vi "home page.vi"() -> ()   [LabVIEW 2019]
uses:
  <vilib>/vision/Image Controls.llb/IMAQ Image.ctl
  <vilib>/Utility/NIReport.llb/Report Type.ctl
  <vilib>/addons/database/Connection.llb/DB Tools Open Connec (String).vi
  <vilib>/addons/_office/excel.llb/Excel Easy Table (str).vi
  <vilib>/measure/mamon.llb/Trigger Detection for 1 Channel.vi
  <vilib>/Utility/NIReport.llb/NI_report.lvclass
  defectsWrapper/defectsWrapper.lvlib
  <vilib>/vision/NI_Vision_Development_Module.lvlib
  <vilib>/vision/driver/NI_Vision_Acquisition_Software.lvlib
  <vilib>/userDefined/High Color/IMAQdx.ctl
  <vilib>/Utility/error.llb/DialogType.ctl
  <vilib>/addons/_office/NI_ReportGenerationToolkit.lvlib
  <vilib>/Utility/NIReport.llb/NI_ReportGenerationCore.lvlib
  <vilib>/measure/NI_MAPro.lvlib
  <vilib>/addons/database/NI_Database_API.lvlib
panel:
  out "sensor thr array":dbl[](array[numeric])
  out "info array":dbl[][](array[numeric])
  out "process error out  2":errorcluster
  out "nan error num":i32
  out "alarm error":errorcluster
  out "sensor error out":errorcluster
  out "img show error":errorcluster
  out "query error in":errorcluster
  out "camera error out":errorcluster
  out "sensor error in":errorcluster
  out "rotate array":errorcluster[](array[cluster])
  out "camera error in":errorcluster
  out "calibration error":errorcluster
  out "rotate error":errorcluster
  out "all errors":errorcluster
  out "DB days to save":i16
  out "orgin data":dbl[](array[numeric])
  out "last difrence":i16
  out "stop ok 2":bool caption="OK"
  out "Overal CURV avg(mm)":dbl format="%#_2g"
  out "Debounce Time":dbl
  out "Frame False Thr":dbl
  out "Col Curves":dbl[](array[numeric])
  out "bottum loop stop":bool
  out "coloumn count stop":bool
  out "query stop":bool=TRUE
  out "alarm loop stop":bool=TRUE
  out "setting stop":bool
  out "rotate stop":bool=TRUE
  out "selected pallet stop":bool
  out "database name":string
  out "denois level array":dbl[](array[numeric])
  out "falling level thr":dbl=59000.0 format="%#_13g"
  out "rotate":bool=TRUE
  out "sen plt indx":i32
  out "snap img":T1
  out "Proc":bool
  out "Frm False":bool
  out "Run/Stop":bool
  out "Sync":bool
  out "Speed (m/min)":string="0"
  out "PLT NUM :":string="1"
  out "avg data array":dbl[](array[numeric])
  out "curv sw info":dbl[](array[numeric])
  out "stop ok":bool caption="OK"
  out "stop live view":bool
  out "stop tab control":bool
  out "dis plt number":i32=45
  out "Tabe name":string="pallet"
  out "PLT NUM":i16
  out "time&date 2":string="08:00:00"
  out "time&date":string="2020/11/22"
  in  "Home":bool
  out "Plt Count":bool
  out "Col. Count":bool
  in  "Sequence Button":bool
  in  "setting":bool
  in  "Graph Button":bool
  in  "report":bool
  in  "stop 3":bool
  out "DPIS":string="DPIS"
  out "capture or not?":bool=TRUE
  out "ready":bool
  out "capture triger":bool
  out "sensor counter":bool
  out "alarm edge":bool
  out "alarm":bool
  out "BoolText.Text":string
  out "counting role":T2(ring)
  out "ch sw sensor2":dbl
  out "ch sw sensor1":dbl
  out "ch sensor3":dbl
  out "ch sensor2":dbl
  out "ch sensor1":dbl
  out "timout":u32=50
  out "Remote Port":u16=502
  out "IP #":string="192.168.88.7"
  out "threshoulds":dbl[](array[numeric])=[900.0, 1000.0, 1600.0, 2400.0, 3000.0, 3000.0]
  out "1st thr":dbl=25.0
  out "2nd thr":dbl=50.0
  out "1st sensor thr":u32=26500
  out "2nd sensor thr":u16=30000
  out "3rd sensor thr":u16=30000
  out "size":dbl=5.0
  out "path image":path
  in  "Button":bool
  out "initilized array":i16[](array[numeric])
  out "Tab Control":enum32{"Page 1", "Page 2", "Page 3"}(tab)
  in  "capture":bool
  out "speed 2":dbl
  out "DEF Type":dbl format="%#.1g"
  out "Sen Plt\nNUM":i16
  out "CURV (mm)":dbl format="%#_3g"
  out "GB defects%":dbl format="%#.1g"
  out "Alarm":bool
  in  "OFF":bool
  out "Pallet Defects View":T1(plugin-control)
  out "GB sit":u32(colorbox)=16448250
  out "curv sit":bool
  out "SWR 2":bool
  out "SWL 2":bool
  in  "Refresh Button":bool
  in  "PLT NUM SYNC":i16
  out "Col\n NUM":dbl format="%#.1g"
  out "Live View":T1(plugin-control)
  out "Col5 CURV(mm)":dbl format="%#_2g"
  out "Sensor Pallet NUM":i16
  out "SideWall Sensors Graph":dynamicdata(graph)=[{"t0"=timestamp(3688782360.9322495 s since 1904-01-01), "dt"=1.0, "Y"=[6594.0]}, {"t0"=timestamp(3688782360.9322495 s since 1904-01-01), "dt"=1.0, "Y"=[65535.0]}]
  out "Col1 CURV(mm)":dbl format="%#_2g"
  out "Col2 CURV(mm)":dbl format="%#_2g"
  out "Col3 CURV(mm)":dbl format="%#_2g"
  out "Col4 CURV(mm)":dbl format="%#_2g"
  out "Overal CURV(mm)":dbl format="%#_2g"
  out "Curvness Sensors Graph":dynamicdata(graph)
  in  "Search Button 2":bool
  in  "Save As Button 2":bool
  in  "pallet sit sel":bool
  in  "swl sel":bool
  in  "swr sel":bool
  in  "PALLET SITUATION":u16(ring) items=["Normal", "Warning", "Error"]
  in  "SWL":u16(ring) items=["Normal", "Error"]
  in  "SWR":u16(ring) items=["Normal", "Error"]
  in  "curv sit sel":bool
  in  "CURV SITUATION":u16(ring) items=["Normal", "Error"]
  in  "def type sel":bool
  in  "DEFECTS TYPE":u16(ring) items=["1", "2"]
  in  "GB_sit sel":bool
  in  "GB SITUATION":u16(ring) items=["Normal", "Warning", "Error"]
  in  "UNTIL":timestamp format="%<%X\n%x>T"
  in  "FROM":timestamp format="%<%X\n%x>T"
  in  "plt num sel":bool
  in  "PALLET NUMBER":dbl
  in  "time sel":bool=TRUE
  in  "TIME":u16(ring)=4 items=["Selected Period", "Last Day", "Last Week", "Last Mounth", "Last Turn"]
  out "Table":string[][](table)
  in  "Base Path":path=path "C:/excel files"
  out "bottum array":bool[](array[boolean])
  out "bottum refrence":refnum<vi>[](array[refnum])
  out "bt ref array":refnum<vi>[](array[refnum])
  in  "117":bool
  in  "118":bool
  in  "119":bool
  in  "120":bool
  in  "121":bool
  in  "122":bool
  in  "123":bool
  in  "124":bool
  in  "125":bool
  in  "126":bool
  in  "127":bool
  in  "128":bool
  in  "129":bool
  in  "130":bool
  in  "131":bool
  in  "132":bool
  in  "133":bool
  in  "134":bool
  in  "135":bool
  in  "136":bool
  in  "137":bool
  in  "138":bool
  in  "139":bool
  in  "140":bool
  in  "141":bool
  in  "142":bool
  in  "143":bool
  in  "144":bool
  in  "145":bool
  in  "146":bool
  in  "147":bool
  in  "148":bool
  in  "149":bool
  in  "150":bool
  in  "151":bool
  in  "152":bool
  in  "153":bool
  in  "154":bool
  in  "155":bool
  in  "156":bool
  in  "157":bool
  in  "158":bool
  in  "159":bool
  in  "160":bool
  in  "161":bool
  in  "162":bool
  in  "163":bool
  in  "164":bool
  in  "165":bool
  in  "166":bool
  in  "167":bool
  in  "168":bool
  in  "169":bool
  in  "170":bool
  in  "171":bool
  in  "172":bool
  in  "173":bool
  in  "174":bool
  in  "175":bool
  in  "176":bool
  in  "177":bool
  in  "178":bool
  in  "179":bool
  in  "180":bool
  in  "181":bool
  in  "182":bool
  in  "183":bool
  in  "184":bool
  in  "185":bool
  in  "186":bool
  in  "187":bool
  in  "188":bool
  in  "189":bool
  in  "190":bool
  in  "191":bool
  in  "192":bool
  in  "193":bool
  in  "194":bool
  in  "195":bool
  in  "196":bool
  in  "197":bool
  in  "198":bool
  in  "199":bool
  in  "200":bool
  in  "201":bool
  in  "202":bool
  in  "203":bool
  in  "204":bool
  in  "205":bool
  in  "206":bool
  in  "207":bool
  in  "208":bool
  in  "209":bool
  in  "210":bool
  in  "211":bool
  in  "212":bool
  in  "213":bool
  in  "214":bool
  in  "215":bool
  in  "216":bool
  in  "217":bool
  in  "218":bool
  in  "219":bool
  in  "220":bool
  in  "221":bool
  in  "222":bool
  in  "223":bool
  in  "224":bool
  in  "225":bool
  in  "226":bool
  in  "227":bool
  in  "228":bool
  in  "229":bool
  in  "230":bool
  in  "231":bool
  in  "232":bool
  in  "116":bool
  in  "115":bool
  in  "114":bool
  in  "113":bool
  in  "112":bool
  in  "111":bool
  in  "110":bool
  in  "109":bool
  in  "108":bool
  in  "107":bool
  in  "106":bool
  in  "105":bool
  in  "104":bool
  in  "103":bool
  in  "102":bool
  in  "101":bool
  in  "100":bool
  in  "99":bool
  in  "98":bool
  in  "97":bool
  in  "96":bool
  in  "95":bool
  in  "94":bool
  in  "93":bool
  in  "92":bool
  in  "91":bool
  in  "90":bool
  in  "89":bool
  in  "88":bool
  in  "87":bool
  in  "86":bool
  in  "85":bool
  in  "84":bool
  in  "83":bool
  in  "82":bool
  in  "81":bool
  in  "80":bool
  in  "79":bool
  in  "78":bool
  in  "77":bool
  in  "76":bool
  in  "75":bool
  in  "74":bool
  in  "73":bool
  in  "72":bool
  in  "71":bool
  in  "70":bool
  in  "69":bool
  in  "68":bool
  in  "67":bool
  in  "66":bool
  in  "65":bool
  in  "64":bool
  in  "63":bool
  in  "62":bool
  in  "61":bool
  in  "60":bool
  in  "59":bool
  in  "58":bool
  in  "57":bool
  in  "56":bool
  in  "55":bool
  in  "54":bool
  in  "53":bool
  in  "52":bool
  in  "51":bool
  in  "50":bool
  in  "49":bool
  in  "48":bool
  in  "47":bool
  in  "46":bool
  in  "45":bool
  in  "44":bool
  in  "43":bool
  in  "42":bool
  in  "41":bool
  in  "40":bool
  in  "39":bool
  in  "38":bool
  in  "37":bool
  in  "36":bool
  in  "35":bool
  in  "34":bool
  in  "33":bool
  in  "32":bool
  in  "31":bool
  in  "30":bool
  in  "29":bool
  in  "28":bool
  in  "27":bool
  in  "26":bool
  in  "25":bool
  in  "24":bool
  in  "23":bool
  in  "22":bool
  in  "21":bool
  in  "20":bool
  in  "19":bool
  in  "18":bool
  in  "17":bool
  in  "16":bool
  in  "15":bool
  in  "14":bool
  in  "13":bool
  in  "12":bool
  in  "11":bool
  in  "10":bool
  in  "9":bool
  in  "8":bool
  in  "7":bool
  in  "6":bool
  in  "5":bool
  in  "4":bool
  in  "3":bool
  in  "2":bool
  in  "1":bool
types:
  T1 = typedef "IMAQ Image.ctl" = refnum<image>
  T2 = enum16{"1st sensor", "2nd sensor", "3rd sensor", "1st+2nd", "1st+3rd", "2nd+3rd", "1st+2nd+3rd"}
  T3 = typedef "Image Type" = u32
  T4 = typedef "IMAQdx.ctl" = refnum<k21>
  T5 = typedef "DialogType.ctl" = u16
  T6 = enum8{"Enabled", "Disabled", "Disabled and Grayed Out"}
  T7 = typedef "NI_Database_API.lvlib/Conn ObjectReference.ctl" = refnum<k1>
  T8 = cluster{"ch sensor1":dbl, "ch sensor2":dbl, "ch sensor3":dbl, "ch sw sensor1":dbl, "ch sw sensor2":dbl}
  T9 = enum32{"Invalid", "Standard", "Closed", "Hidden", "Minimized", "Maximized"}
  T10 = cluster{"ch sensor1":dbl, "ch sensor2":dbl, "chs ensor3":dbl, "ch sw sensor1":dbl, "ch sw sensor2":dbl}
  T11 = cluster{"level1 thr":dbl, "level2 thr":dbl, "gr.th1":dbl, "gr.th2":dbl, "gr.th3":dbl, "gr.th4":dbl, "gr.th5":dbl, "gr.th6":dbl, "gr.th7":dbl, "gr.th8":dbl, "gr.th9":dbl, "def size":dbl, "Frame False Thr":dbl}
  T12 = cluster{"Thr1":dbl, "Thr2":dbl, "Thr3":dbl, "Port":dbl, "time out":dbl, "SWR thr":dbl, "SWL thr ":dbl, "Curv thr (mm)":dbl, "SW timout(s)":dbl, "falling level thr":dbl, "denoise thr1":dbl, "denoise thr2":dbl, "denoise thr3":dbl, "low level read thr":dbl, "Debounce Time":dbl}
  T13 = cluster{"plt number dis":i16, "Table Name":string, "Database Name":string, "DB days to save":i16}
  T14 = enum16{"maximized", "minimized", "normal", "no change"}
  T15 = typedef "NI_ReportGenerationCore.lvlib/Report Type.ctl" = enum16{"HTML", "Word", "Excel"}
  T16 = typedef "LVDateTimeRec.ctl" = cluster{"fractional second":dbl, "second":i32, "minute":i32, "hour":i32, "day of month":i32, "month":i32, "year":i32, "day of week":i32, "day of year":i32, "DST":i32}
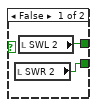
[diagram p6: hidden frame]
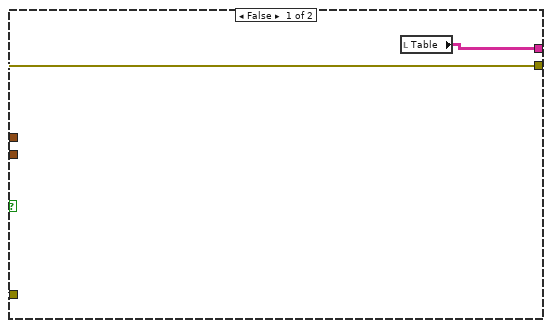
[diagram p8: hidden frame]
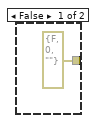
[diagram p10: hidden frame]
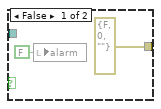
[diagram p11: hidden frame]
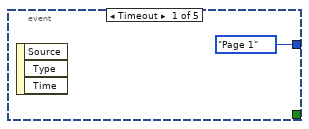
[diagram p14: hidden frame]
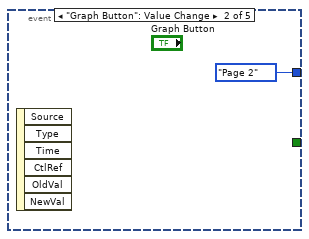
[diagram p15: hidden frame]
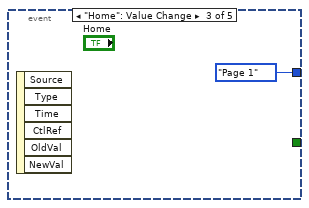
[diagram p16: hidden frame]
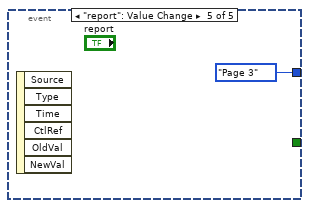
[diagram p17: hidden frame]
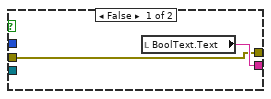
[diagram p19: hidden frame]
diagram:
  w26 = 2 ("dimension size")
  w21 = 100 ("dimension size")
  (unwired) FALSE ("process")
  w67 = FALSE ("nan error")
  w68 = 0.0
  w75 = FALSE
  w100 = T3 4 items=["Grayscale (U8)", "Grayscale (I16)", "Grayscale (SGL)", "Complex (CSG)", "RGB (U32)", "HSL (U32)", "RGB (U64)", "Grayscale (U16)"] ("Image Type")
  n1 = call "load Defects Script.vi"() -> ()  [unwired: 11 in, 1 out]
  n2 = while {
    tunnel: [w345] -> w62
    stop <- w345 stop-if-true
    n3 = Wait (ms)(milliseconds to wait=u32 5) -> ()  [unwired: 1 out]
    n4 = local read "stop ok"() -> (w345:bool)
    n5 = Build Array("232", "231", "230", "229", "228", "227", "226", "225", "224", "223", "222", "221", "220", "219", "218", "217", "216", "215", "214", "213", "212", "211", "210", "209", "208", "207", "206", "205", "204", "203", "202", "201", "200", "199", "198", "197", "196", "195", "194", "193", "192", "191", "190", "189", "188", "187", "186", "185", "184", "183", "182", "181", "180", "179", "178", "177", "176", "175", "174", "173", "172", "171", "170", "169", "168", "167", "166", "165", "164", "163", "162", "161", "160", "159", "158", "157", "156", "155", "154", "153", "152", "151", "150", "149", "148", "147", "146", "145", "144", "143", "142", "141", "140", "139", "138", "137", "136", "135", "134", "133", "132", "131", "130", "129", "128", "127", "126", "125", "124", "123", "122", "121", "120", "119", "118", "117", "116", "115", "114", "113", "112", "111", "110", "109", "108", "107", "106", "105", "104", "103", "102", "101", "100", "99", "98", "97", "96", "95", "94", "93", "92", "91", "90", "89", "88", "87", "86", "85", "84", "83", "82", "81", "80", "79", "78", "77", "76", "75", "74", "73", "72", "71", "70", "69", "68", "67", "66", "65", "64", "63", "62", "61", "60", "59", "58", "57", "56", "55", "54", "53", "52", "51", "50", "49", "48", "47", "46", "45", "44", "43", "42", "41", "40", "39", "38", "37", "36", "35", "34", "33", "32", "31", "30", "29", "28", "27", "26", "25", "24", "23", "22", "21", "20", "19", "18", "17", "16", "15", "14", "13", "12", "11", "10", "9", "8", "7", "6", "5", "4", "3", "2", "1") -> (→"bottum array":bool[])
  }
  "bottum loop stop" <- w62
  n6 = control-ref of="232"() -> (w344:refnum<vi>)
  n7 = control-ref of="231"() -> (w343:refnum<vi>)
  n8 = control-ref of="230"() -> (w342:refnum<vi>)
  n9 = control-ref of="229"() -> (w341:refnum<vi>)
  n10 = control-ref of="228"() -> (w340:refnum<vi>)
  n11 = control-ref of="227"() -> (w339:refnum<vi>)
  n12 = control-ref of="226"() -> (w338:refnum<vi>)
  n13 = control-ref of="225"() -> (w337:refnum<vi>)
  n14 = control-ref of="224"() -> (w336:refnum<vi>)
  n15 = control-ref of="223"() -> (w335:refnum<vi>)
  n16 = control-ref of="222"() -> (w334:refnum<vi>)
  n17 = control-ref of="221"() -> (w333:refnum<vi>)
  n18 = control-ref of="220"() -> (w332:refnum<vi>)
  n19 = control-ref of="219"() -> (w331:refnum<vi>)
  n20 = control-ref of="218"() -> (w330:refnum<vi>)
  n21 = control-ref of="217"() -> (w329:refnum<vi>)
  n22 = control-ref of="216"() -> (w328:refnum<vi>)
  n23 = control-ref of="215"() -> (w327:refnum<vi>)
  n24 = control-ref of="214"() -> (w326:refnum<vi>)
  n25 = control-ref of="213"() -> (w325:refnum<vi>)
  n26 = control-ref of="212"() -> (w324:refnum<vi>)
  n27 = control-ref of="211"() -> (w323:refnum<vi>)
  n28 = control-ref of="210"() -> (w322:refnum<vi>)
  n29 = control-ref of="209"() -> (w321:refnum<vi>)
  n30 = control-ref of="208"() -> (w320:refnum<vi>)
  n31 = control-ref of="207"() -> (w319:refnum<vi>)
  n32 = control-ref of="206"() -> (w318:refnum<vi>)
  n33 = control-ref of="205"() -> (w317:refnum<vi>)
  n34 = control-ref of="204"() -> (w316:refnum<vi>)
  n35 = control-ref of="203"() -> (w315:refnum<vi>)
  n36 = control-ref of="202"() -> (w314:refnum<vi>)
  n37 = control-ref of="201"() -> (w313:refnum<vi>)
  n38 = control-ref of="200"() -> (w312:refnum<vi>)
  n39 = control-ref of="199"() -> (w311:refnum<vi>)
  n40 = control-ref of="198"() -> (w310:refnum<vi>)
  n41 = control-ref of="197"() -> (w309:refnum<vi>)
  n42 = control-ref of="196"() -> (w308:refnum<vi>)
  n43 = control-ref of="195"() -> (w307:refnum<vi>)
  n44 = control-ref of="194"() -> (w306:refnum<vi>)
  n45 = control-ref of="193"() -> (w305:refnum<vi>)
  n46 = control-ref of="192"() -> (w304:refnum<vi>)
  n47 = control-ref of="191"() -> (w303:refnum<vi>)
  n48 = control-ref of="190"() -> (w302:refnum<vi>)
  n49 = control-ref of="189"() -> (w301:refnum<vi>)
  n50 = control-ref of="188"() -> (w300:refnum<vi>)
  n51 = control-ref of="187"() -> (w299:refnum<vi>)
  n52 = control-ref of="186"() -> (w298:refnum<vi>)
  n53 = control-ref of="185"() -> (w297:refnum<vi>)
  n54 = control-ref of="184"() -> (w296:refnum<vi>)
  n55 = control-ref of="183"() -> (w295:refnum<vi>)
  n56 = control-ref of="182"() -> (w294:refnum<vi>)
  n57 = control-ref of="181"() -> (w293:refnum<vi>)
  n58 = control-ref of="180"() -> (w292:refnum<vi>)
  n59 = control-ref of="179"() -> (w291:refnum<vi>)
  n60 = control-ref of="178"() -> (w290:refnum<vi>)
  n61 = control-ref of="177"() -> (w289:refnum<vi>)
  n62 = control-ref of="176"() -> (w288:refnum<vi>)
  n63 = control-ref of="175"() -> (w287:refnum<vi>)
  n64 = control-ref of="174"() -> (w286:refnum<vi>)
  n65 = control-ref of="173"() -> (w285:refnum<vi>)
  n66 = control-ref of="172"() -> (w284:refnum<vi>)
  n67 = control-ref of="171"() -> (w283:refnum<vi>)
  n68 = control-ref of="170"() -> (w282:refnum<vi>)
  n69 = control-ref of="169"() -> (w281:refnum<vi>)
  n70 = control-ref of="168"() -> (w280:refnum<vi>)
  n71 = control-ref of="167"() -> (w279:refnum<vi>)
  n72 = control-ref of="166"() -> (w278:refnum<vi>)
  n73 = control-ref of="165"() -> (w277:refnum<vi>)
  n74 = control-ref of="164"() -> (w276:refnum<vi>)
  n75 = control-ref of="163"() -> (w275:refnum<vi>)
  n76 = control-ref of="162"() -> (w274:refnum<vi>)
  n77 = control-ref of="161"() -> (w273:refnum<vi>)
  n78 = control-ref of="160"() -> (w272:refnum<vi>)
  n79 = control-ref of="159"() -> (w271:refnum<vi>)
  n80 = control-ref of="158"() -> (w270:refnum<vi>)
  n81 = control-ref of="157"() -> (w269:refnum<vi>)
  n82 = control-ref of="156"() -> (w268:refnum<vi>)
  n83 = control-ref of="155"() -> (w267:refnum<vi>)
  n84 = control-ref of="154"() -> (w266:refnum<vi>)
  n85 = control-ref of="153"() -> (w265:refnum<vi>)
  n86 = control-ref of="152"() -> (w264:refnum<vi>)
  n87 = control-ref of="151"() -> (w263:refnum<vi>)
  n88 = control-ref of="150"() -> (w262:refnum<vi>)
  n89 = control-ref of="149"() -> (w261:refnum<vi>)
  n90 = control-ref of="148"() -> (w260:refnum<vi>)
  n91 = control-ref of="147"() -> (w259:refnum<vi>)
  n92 = control-ref of="146"() -> (w258:refnum<vi>)
  n93 = control-ref of="145"() -> (w257:refnum<vi>)
  n94 = control-ref of="144"() -> (w256:refnum<vi>)
  n95 = control-ref of="143"() -> (w255:refnum<vi>)
  n96 = control-ref of="142"() -> (w254:refnum<vi>)
  n97 = control-ref of="141"() -> (w253:refnum<vi>)
  n98 = control-ref of="140"() -> (w252:refnum<vi>)
  n99 = control-ref of="139"() -> (w251:refnum<vi>)
  n100 = control-ref of="138"() -> (w250:refnum<vi>)
  n101 = control-ref of="137"() -> (w249:refnum<vi>)
  n102 = control-ref of="136"() -> (w248:refnum<vi>)
  n103 = control-ref of="135"() -> (w247:refnum<vi>)
  n104 = control-ref of="134"() -> (w246:refnum<vi>)
  n105 = control-ref of="133"() -> (w245:refnum<vi>)
  n106 = control-ref of="132"() -> (w244:refnum<vi>)
  n107 = control-ref of="131"() -> (w243:refnum<vi>)
  n108 = control-ref of="130"() -> (w242:refnum<vi>)
  n109 = control-ref of="129"() -> (w241:refnum<vi>)
  n110 = control-ref of="128"() -> (w240:refnum<vi>)
  n111 = control-ref of="127"() -> (w239:refnum<vi>)
  n112 = control-ref of="126"() -> (w238:refnum<vi>)
  n113 = control-ref of="125"() -> (w237:refnum<vi>)
  n114 = control-ref of="124"() -> (w236:refnum<vi>)
  n115 = control-ref of="123"() -> (w235:refnum<vi>)
  n116 = control-ref of="122"() -> (w234:refnum<vi>)
  n117 = control-ref of="121"() -> (w233:refnum<vi>)
  n118 = control-ref of="120"() -> (w232:refnum<vi>)
  n119 = control-ref of="119"() -> (w231:refnum<vi>)
  n120 = control-ref of="118"() -> (w230:refnum<vi>)
  n121 = control-ref of="117"() -> (w229:refnum<vi>)
  n122 = control-ref of="116"() -> (w228:refnum<vi>)
  n123 = control-ref of="115"() -> (w227:refnum<vi>)
  n124 = control-ref of="114"() -> (w226:refnum<vi>)
  n125 = control-ref of="113"() -> (w225:refnum<vi>)
  n126 = control-ref of="112"() -> (w224:refnum<vi>)
  n127 = control-ref of="111"() -> (w223:refnum<vi>)
  n128 = control-ref of="110"() -> (w222:refnum<vi>)
  n129 = control-ref of="109"() -> (w221:refnum<vi>)
  n130 = control-ref of="108"() -> (w220:refnum<vi>)
  n131 = control-ref of="107"() -> (w219:refnum<vi>)
  n132 = control-ref of="106"() -> (w218:refnum<vi>)
  n133 = control-ref of="105"() -> (w217:refnum<vi>)
  n134 = control-ref of="104"() -> (w216:refnum<vi>)
  n135 = control-ref of="103"() -> (w215:refnum<vi>)
  n136 = control-ref of="102"() -> (w214:refnum<vi>)
  n137 = control-ref of="101"() -> (w213:refnum<vi>)
  n138 = control-ref of="100"() -> (w212:refnum<vi>)
  n139 = control-ref of="99"() -> (w211:refnum<vi>)
  n140 = control-ref of="98"() -> (w210:refnum<vi>)
  n141 = control-ref of="97"() -> (w209:refnum<vi>)
  n142 = control-ref of="96"() -> (w208:refnum<vi>)
  n143 = control-ref of="95"() -> (w207:refnum<vi>)
  n144 = control-ref of="94"() -> (w206:refnum<vi>)
  n145 = control-ref of="93"() -> (w205:refnum<vi>)
  n146 = control-ref of="92"() -> (w204:refnum<vi>)
  n147 = control-ref of="91"() -> (w203:refnum<vi>)
  n148 = control-ref of="90"() -> (w202:refnum<vi>)
  n149 = control-ref of="89"() -> (w201:refnum<vi>)
  n150 = control-ref of="88"() -> (w200:refnum<vi>)
  n151 = control-ref of="87"() -> (w199:refnum<vi>)
  n152 = control-ref of="86"() -> (w198:refnum<vi>)
  n153 = control-ref of="85"() -> (w197:refnum<vi>)
  n154 = control-ref of="84"() -> (w196:refnum<vi>)
  n155 = control-ref of="83"() -> (w195:refnum<vi>)
  n156 = control-ref of="82"() -> (w194:refnum<vi>)
  n157 = control-ref of="81"() -> (w193:refnum<vi>)
  n158 = control-ref of="80"() -> (w192:refnum<vi>)
  n159 = control-ref of="79"() -> (w191:refnum<vi>)
  n160 = control-ref of="78"() -> (w190:refnum<vi>)
  n161 = control-ref of="77"() -> (w189:refnum<vi>)
  n162 = control-ref of="76"() -> (w188:refnum<vi>)
  n163 = control-ref of="75"() -> (w187:refnum<vi>)
  n164 = control-ref of="74"() -> (w186:refnum<vi>)
  n165 = control-ref of="73"() -> (w185:refnum<vi>)
  n166 = control-ref of="72"() -> (w184:refnum<vi>)
  n167 = control-ref of="71"() -> (w183:refnum<vi>)
  n168 = control-ref of="70"() -> (w182:refnum<vi>)
  n169 = control-ref of="69"() -> (w181:refnum<vi>)
  n170 = control-ref of="68"() -> (w180:refnum<vi>)
  n171 = control-ref of="67"() -> (w179:refnum<vi>)
  n172 = control-ref of="66"() -> (w178:refnum<vi>)
  n173 = control-ref of="65"() -> (w177:refnum<vi>)
  n174 = control-ref of="64"() -> (w176:refnum<vi>)
  n175 = control-ref of="63"() -> (w175:refnum<vi>)
  n176 = control-ref of="62"() -> (w174:refnum<vi>)
  n177 = control-ref of="61"() -> (w173:refnum<vi>)
  n178 = control-ref of="60"() -> (w172:refnum<vi>)
  n179 = control-ref of="59"() -> (w171:refnum<vi>)
  n180 = local write "capture or not?"(w67) -> ()
  n181 = local write "stop ok"(w67) -> ()
  n182 = local write "alarm"(w67) -> ()
  n183 = property on="Alarm" class="Bool (strict)"() -> ("Colors [4]"=w98:cluster{u32, u32}[])  [unwired: 2 in, 2 out]
  n184 = control-ref of="58"() -> (w170:refnum<vi>)
  n185 = control-ref of="57"() -> (w169:refnum<vi>)
  n186 = control-ref of="56"() -> (w168:refnum<vi>)
  n187 = control-ref of="55"() -> (w167:refnum<vi>)
  n188 = control-ref of="54"() -> (w166:refnum<vi>)
  n189 = control-ref of="53"() -> (w165:refnum<vi>)
  n190 = control-ref of="52"() -> (w164:refnum<vi>)
  n191 = control-ref of="51"() -> (w163:refnum<vi>)
  n192 = control-ref of="50"() -> (w162:refnum<vi>)
  n193 = control-ref of="49"() -> (w161:refnum<vi>)
  n194 = control-ref of="48"() -> (w160:refnum<vi>)
  n195 = control-ref of="47"() -> (w159:refnum<vi>)
  n196 = control-ref of="46"() -> (w158:refnum<vi>)
  n197 = control-ref of="45"() -> (w157:refnum<vi>)
  n198 = control-ref of="44"() -> (w156:refnum<vi>)
  n199 = control-ref of="43"() -> (w155:refnum<vi>)
  n200 = control-ref of="42"() -> (w154:refnum<vi>)
  n201 = control-ref of="41"() -> (w153:refnum<vi>)
  n202 = control-ref of="40"() -> (w152:refnum<vi>)
  n203 = control-ref of="39"() -> (w151:refnum<vi>)
  n204 = control-ref of="38"() -> (w150:refnum<vi>)
  n205 = control-ref of="37"() -> (w149:refnum<vi>)
  n206 = control-ref of="36"() -> (w148:refnum<vi>)
  n207 = control-ref of="35"() -> (w147:refnum<vi>)
  n208 = control-ref of="34"() -> (w146:refnum<vi>)
  n209 = control-ref of="33"() -> (w145:refnum<vi>)
  n210 = control-ref of="32"() -> (w144:refnum<vi>)
  n211 = control-ref of="31"() -> (w143:refnum<vi>)
  n212 = control-ref of="30"() -> (w142:refnum<vi>)
  n213 = control-ref of="29"() -> (w141:refnum<vi>)
  n214 = control-ref of="28"() -> (w140:refnum<vi>)
  n215 = control-ref of="27"() -> (w139:refnum<vi>)
  n216 = control-ref of="26"() -> (w138:refnum<vi>)
  n217 = control-ref of="25"() -> (w137:refnum<vi>)
  n218 = control-ref of="24"() -> (w136:refnum<vi>)
  n219 = control-ref of="23"() -> (w135:refnum<vi>)
  n220 = control-ref of="22"() -> (w134:refnum<vi>)
  n221 = control-ref of="21"() -> (w133:refnum<vi>)
  n222 = control-ref of="20"() -> (w132:refnum<vi>)
  n223 = control-ref of="19"() -> (w131:refnum<vi>)
  n224 = control-ref of="18"() -> (w130:refnum<vi>)
  n225 = control-ref of="17"() -> (w129:refnum<vi>)
  n226 = control-ref of="16"() -> (w128:refnum<vi>)
  n227 = control-ref of="15"() -> (w127:refnum<vi>)
  n228 = control-ref of="14"() -> (w126:refnum<vi>)
  n229 = control-ref of="13"() -> (w125:refnum<vi>)
  n230 = control-ref of="12"() -> (w124:refnum<vi>)
  n231 = control-ref of="11"() -> (w123:refnum<vi>)
  n232 = control-ref of="10"() -> (w122:refnum<vi>)
  n233 = control-ref of="9"() -> (w121:refnum<vi>)
  n234 = control-ref of="8"() -> (w120:refnum<vi>)
  n235 = control-ref of="7"() -> (w119:refnum<vi>)
  n236 = control-ref of="6"() -> (w118:refnum<vi>)
  n237 = control-ref of="5"() -> (w117:refnum<vi>)
  n238 = control-ref of="4"() -> (w116:refnum<vi>)
  n239 = control-ref of="3"() -> (w115:refnum<vi>)
  n240 = control-ref of="2"() -> (w114:refnum<vi>)
  n241 = control-ref of="1"() -> (w113:refnum<vi>)
  n242 = Replace Array Subset(array=w98, new element=cluster{u32, u32} {16448250, 16448250} ("new element/subarray"), index=0) -> (w96:cluster{u32, u32}[])
  n243 = property on="PLT NUM SYNC" class="DigNum (strict)"("Value"=i16 1 ("PLT NUM SYNC")) -> ()  [unwired: 2 in, 2 out]
  n244 = property on="Sen Plt\nNUM" class="DigNum (strict)"("Value"=i16 0 ("Sen Plt\nNUM")) -> ()  [unwired: 2 in, 2 out]
  n245 = property on="GB sit" class="ColBox"("Value"=u32 16448250 ("GB sit")) -> ()  [unwired: 2 in, 2 out]
  n246 = property on="Sensor Pallet NUM" class="DigNum (strict)"("Value"=i16 0 ("Sensor Pallet NUM")) -> ()  [unwired: 2 in, 2 out]
  n247 = property on="Alarm" class="Bool (strict)"("Colors [4]"=w96) -> ()  [unwired: 2 in, 2 out]
  n248 = property on="Col. Count" class="Bool (strict)"("Value"=w75) -> ()  [unwired: 2 in, 2 out]
  n249 = property on="Plt Count" class="Bool (strict)"("Value"=w75) -> ()  [unwired: 2 in, 2 out]
  n250 = property on="Run/Stop" class="Bool (strict)"("Value"=w75) -> ()  [unwired: 2 in, 2 out]
  n251 = property on="curv sit" class="Bool (strict)"("Value"=FALSE ("curv sit")) -> ()  [unwired: 2 in, 2 out]
  n252 = property on="Table" class="Tbl (strict)"("Column Headers[]"=string[] ["PLT_NUM", "DATE_TIME", "GB_DEF", "DEF_TYPE", "GB_SIT", "CURV", "CURV_SIT", "SWR", "SWL", "PLT_SIT", "COL1 CURV", "COL2 CURV", "COL3 CURV", "COL4 CURV", "COL5 CURV"] ("Column Header Strings[]")) -> ()  [unwired: 2 in, 2 out]
  n253 = property on="CURV (mm)" class="DigNum (strict)"("Value"=0.0 ("CURV (mm)")) -> ()  [unwired: 2 in, 2 out]
  n254 = property on="GB defects%" class="DigNum (strict)"("Value"=0.0 ("GB defects%")) -> ()  [unwired: 2 in, 2 out]
  n255 = property on="Speed (m/min)" class="Str"("Value"="0" ("Speed :")) -> ()  [unwired: 2 in, 2 out]
  n256 = property on="time&date 2" class="Str"("Value"="" ("time&date 2")) -> ()  [unwired: 2 in, 2 out]
  n257 = property on="time&date" class="Str"("Value"="" ("time&date")) -> ()  [unwired: 2 in, 2 out]
  n258 = property on="PLT NUM :" class="Str"("Value"="1" ("PLT NUM :")) -> ()  [unwired: 2 in, 2 out]
  n259 = property on="Col\n NUM" class="DigNum (strict)"("Value"=0.0 ("Col\n NUM")) -> ()  [unwired: 2 in, 2 out]
  n260 = property on="DEF Type" class="DigNum (strict)"("Value"=1.0 ("DEF Type")) -> ()  [unwired: 2 in, 2 out]
  n261 = property on="Overal CURV avg(mm)" class="DigNum (strict)"("Value"=0.0 ("Overal CURV(mm)")) -> ()  [unwired: 2 in, 2 out]
  n262 = property on="SWR 2" class="Bool (strict)"("Value"=FALSE ("SWR 2")) -> ()  [unwired: 2 in, 2 out]
  n263 = property on="SWL 2" class="Bool (strict)"("Value"=FALSE ("SWL 2")) -> ()  [unwired: 2 in, 2 out]
  n264 = property on="Proc" class="Bool (strict)"("Value"=FALSE ("Proc")) -> ()  [unwired: 2 in, 2 out]
  n265 = property on="Alarm" class="Bool (strict)"("Blinking"=FALSE ("alarm")) -> ()  [unwired: 2 in, 2 out]
  n266 = property on="Sync" class="Bool (strict)"("Value"=FALSE ("Sync")) -> ()  [unwired: 2 in, 2 out]
  n267 = local write "CURV (mm)"(0.0 ("CURV %")) -> ()
  n268 = property on="Col2 CURV(mm)" class="DigNum (strict)"("Value"=w68) -> ()  [unwired: 2 in, 2 out]
  n269 = property on="Col3 CURV(mm)" class="DigNum (strict)"("Value"=w68) -> ()  [unwired: 2 in, 2 out]
  n270 = property on="Col4 CURV(mm)" class="DigNum (strict)"("Value"=w68) -> ()  [unwired: 2 in, 2 out]
  n271 = property on="Col5 CURV(mm)" class="DigNum (strict)"("Value"=w68) -> ()  [unwired: 2 in, 2 out]
  n272 = property on="Col1 CURV(mm)" class="DigNum (strict)"("Value"=w68) -> ()  [unwired: 2 in, 2 out]
  n273 = Build Array(w344, w343, w342, w341, w340, w339, w338, w337, w336, w335, w334, w333, w332, w331, w330, w329, w328, w327, w326, w325, w324, w323, w322, w321, w320, w319, w318, w317, w316, w315, w314, w313, w312, w311, w310, w309, w308, w307, w306, w305, w304, w303, w302, w301, w300, w299, w298, w297, w296, w295, w294, w293, w292, w291, w290, w289, w288, w287, w286, w285, w284, w283, w282, w281, w280, w279, w278, w277, w276, w275, w274, w273, w272, w271, w270, w269, w268, w267, w266, w265, w264, w263, w262, w261, w260, w259, w258, w257, w256, w255, w254, w253, w252, w251, w250, w249, w248, w247, w246, w245, w244, w243, w242, w241, w240, w239, w238, w237, w236, w235, w234, w233, w232, w231, w230, w229, w228, w227, w226, w225, w224, w223, w222, w221, w220, w219, w218, w217, w216, w215, w214, w213, w212, w211, w210, w209, w208, w207, w206, w205, w204, w203, w202, w201, w200, w199, w198, w197, w196, w195, w194, w193, w192, w191, w190, w189, w188, w187, w186, w185, w184, w183, w182, w181, w180, w179, w178, w177, w176, w175, w174, w173, w172, w171, w170, w169, w168, w167, w166, w165, w164, w163, w162, w161, w160, w159, w158, w157, w156, w155, w154, w153, w152, w151, w150, w149, w148, w147, w146, w145, w144, w143, w142, w141, w140, w139, w138, w137, w136, w135, w134, w133, w132, w131, w130, w129, w128, w127, w126, w125, w124, w123, w122, w121, w120, w119, w118, w117, w116, w115, w114, w113) -> (w109:refnum<vi>[])
  "bottum refrence" <- w109
  n274 = disable-structure shown="Disabled" {
    frame Disabled {
      n275 = call "IMAQ Create"("Image Name"="mainimg", "error in (no error)"=errorcluster {"status"=FALSE, "code"=0, "source"=""}) -> ("New Image"=w593:T1, "error out"=w587:errorcluster)  [unwired: 3 in]
      n276 = call "Vision Acquisition2"("error in"=w587) -> ("Image Out"=w585:T1, "error out"=w582:errorcluster)  [unwired: 24 in, 1 out]
      n277 = call "IMAQ Create"("Image Name"="rotate", "error in (no error)"=w582) -> ("New Image"=w583:T1, "error out"=w581:errorcluster)  [unwired: 3 in]
      n278 = while {
        tunnel: w593 -> [w607]
        tunnel: [w612] -> w590
        tunnel: [w598] -> w588
        tunnel: T4 "cam0" ("Session In") -> [w611]
        tunnel: w585 -> [w610]
        tunnel: w583 -> [w608]
        shift-right: [w599] -> w580
        shift-left: w581 -> [w609]
        stop <- w612 stop-if-true
        # "Live view"
        n279 = flat-sequence {
          tunnel: w611 -> [w620]
          tunnel: w610 -> [w619]
          tunnel: w609 -> [w618]
          tunnel: w608 -> [w615]
          tunnel: w607 -> [w614]
          tunnel: [w617] -> w606
          tunnel: [w616] -> w605
          tunnel: [w615] -> w604
          tunnel: [w614] -> w603
          tunnel: w606 -> [w622]
          tunnel: w605 -> [w623]
          tunnel: w604 -> [w627]
          tunnel: w603 -> [w624]
          tunnel: [w627] -> w602
          tunnel: [w626] -> w601
          tunnel: [w621] -> w600
          tunnel: [w621] -> w595
          tunnel: w602 -> [w630]
          tunnel: w601 -> [w632]
          tunnel: w600 -> [w631]
          tunnel: [w633] -> w597
          tunnel: [w629] -> w596
          tunnel: w595 -> [w628]
          tunnel: [w634] -> w598
          tunnel: [w635] -> w599
          tunnel: w596 -> [w634]
          tunnel: w597 -> [w635]
          frame #0 {
            n280 = call <vilib>:"IMAQdx Grab.vi"("error in"=w618, "Image In"=w619, "Session In"=w620) -> ("error out"=w617:errorcluster, "Image Out"=w616:T1)  [unwired: 1 in, 6 out]
          }
          frame #1 {
            n281 = call "IMAQ Rotate"("error in (no error)"=w622, "Angle (degrees)"=sgl 180.0, "Image Dst"=w624, "Image Src"=w623) -> ("error out"=w626:errorcluster, "Image Dst Out"=w621:T1)  [unwired: 6 in]
          }
          frame #2 {
            n282 = call "IMAQ Copy"("error in (no error)"=w632, "Image Dst"=w630, "Image Src"=w631) -> ("error out"=w633:errorcluster, "Image Dst Out"=w629:T1)  [unwired: 3 in]
            "Live View" <- w628
          }
          frame #3 {
            "snap img" <- w634
          }
        }
        n283 = Wait (ms)(milliseconds to wait=u32 20) -> ()  [unwired: 1 out]
        n284 = local read "stop ok"() -> (w612:bool)
        "camera error in" <- w599
      }
      "stop live view" <- w590
      n285 = call "IMAQ Dispose"("All Images? (No)"=TRUE, "Image"=w588, "error in (no error)"=w580) -> ("error out"=→"camera error out":errorcluster)  [unwired: 3 in]
    }
    frame Enabled {
    }
  }
  n286 = Initialize Array(i16 0 ("element"), 232 ("dimension size")) -> (w110:i16[])
  n287 = property on="Frm False" class="Bool (strict)"("Value"=FALSE ("Frm False")) -> ()  [unwired: 2 in, 2 out]
  n288 = disable-structure shown="Disabled" {
    disable-tunnel: [w638 _] -> w37
    disable-tunnel: [w636 _] -> w18
    frame Disabled {
      n289 = while {
        tunnel: [w652] -> w638
        shift-right: [w639] -> w636
        shift-left: errorcluster {"status"=FALSE, "code"=0, "source"=""} ("error in (no error)") -> [w649]
        stop <- w640 stop-if-true
        w645 = T5 0 items=["no dialog", "OK message", "continue or stop message", "OK message + warnings", "continue/stop + warnings"] ("type of dialog (OK msg:1)")
        n290 = Wait (ms)(milliseconds to wait=u32 5) -> ()  [unwired: 1 out]
        n291 = property on="IP #" class="Str"(error in=w649) -> (error out=w648:errorcluster, "Value"=w651:string)  [unwired: 1 in, 1 out]
        n292 = property on="Remote Port" class="DigNum (strict)"(error in=w648) -> (error out=w647:errorcluster, "Value"=w650:u16)  [unwired: 1 in, 1 out]
        n293 = local read "stop ok"() -> (w641:bool)
        n294 = TCP Open Connection(address=w651, remote port or service name=w650, error in (no error)=w647) -> (connection ID=w652:refnum<k5>, error out=w646:errorcluster)  [unwired: 2 in]
        n295 = call <vilib>:"Simple Error Handler.vi"("type of dialog (OK msg:1)"=w645, "error in (no error)"=w646) -> ("error?"=w644:bool, "error out"=w639:errorcluster)  [unwired: 3 in, 3 out]
        n296 = Not(x=w644) -> (.not. x?=w642:bool)
        n297 = Or(x=w642, y=w641) -> (x .or. y?=w640:bool)
      }
    }
    frame Enabled {
    }
  }
  n298 = for {
    tunnel: [w654] -> w105 mode=indexing
    shift-right: [w664] -> _
    shift-left: w110 -> [w665]
    tunnel: w109 -> [w660] mode=indexing
    tunnel: errorcluster {"status"=FALSE, "code"=0, "source"=""} ("error in (no error)") -> [w659]
    tunnel: [w653] -> w107 mode=indexing
    i -> [w663]
    n299 = Replace Array Subset(array=w665, new element=w663, index=w663) -> (w664:i16[])
    "initilized array" <- w664
    n300 = property class="Bool"(reference=w660, error in=w659) -> (reference out=w669:refnum<vi>, error out=w667:errorcluster, "Label.Text"=w668:string)
    n301 = control-ref of="Button"() -> (w662:refnum<vi>)
    n302 = property class="Bool"(reference=w669, error in=w667, "BoolText.Text"=w668) -> (reference out=w657:refnum<vi>, error out=w658:errorcluster)
    n303 = property class="Bool"(reference=w662) -> ("Colors [4]"=w661:cluster{u32, u32}[])  [unwired: 1 in, 2 out]
    n304 = property class="Bool"(reference=w657, error in=w658, "Colors [4]"=w661) -> (reference out=w656:refnum<vi>, error out=w655:errorcluster)
    n305 = property class="Bool"(reference=w656, error in=w655, "DisabledEnum"=T6."Disabled and Grayed Out" ("Disabled")) -> (reference out=w654:refnum<vi>, error out=w653:errorcluster)
  }
  n306 = Initialize Array(0.0 ("element"), w21) -> (w31:dbl[])
  n307 = Initialize Array(0.0 ("element"), w21) -> (w29:dbl[])
  n308 = Initialize Array(0.0 ("element"), w26) -> (w28:dbl[])
  n309 = Initialize Array(0.0 ("element"), w21) -> (w30:dbl[])
  n310 = Initialize Array(0.0 ("element"), w26) -> (w27:dbl[])
  n311 = call-poly <vilib>:"DB Tools Open Connection.vi"("error in (no error)"=errorcluster {"status"=FALSE, "code"=0, "source"=""}, "connection information"="DSGS" ("database name 2")) -> ("error out"=w48:errorcluster, "connection reference"=w47:T7)  [unwired: 6 in]
  n312 = while {
    tunnel: [w674] -> w92
    tunnel: FALSE ("stop 4") -> [w673]
    tunnel: [FALSE ("Sync")] -> w91
    tunnel: [i16 1 ("PLT NUM SYNC")] -> w90
    stop <- w674 stop-if-true
    # "Tab control"
    n313 = event shown="[3] \"stop 3\": Value Change" {
      selector: _ -> [_ _ _ _ _]
      dyn-events: _ -> [_ _ _ _ _]
      timeout: _ -> [_ _ _ _ _]
      tunnel: [enum32{"Page 1", "Page 2", "Page 3"}."Page 1" ("Tab Control") enum32{"Page 1", "Page 2", "Page 3"}."Page 2" ("Tab Control") enum32{"Page 1", "Page 2", "Page 3"}."Page 1" ("Tab Control") w679 enum32{"Page 1", "Page 2", "Page 3"}."Page 3" ("Tab Control")] -> w670
      tunnel: [_ _ _ w680 _] -> w674
      event Timeout {
        n314 = event-data() -> ()  [unwired: 1 in, 3 out]
      }
      event "Graph Button": Value Change {
        n315 = event-data() -> ()  [unwired: 1 in, 6 out]
      }
      event "Home": Value Change {
        n316 = event-data() -> ()  [unwired: 1 in, 6 out]
      }
      event "stop 3": Value Change {
        n317 = event-data() -> ()  [unwired: 1 in, 6 out]
        n318 = call "close.vi"("Enable"="stop 3") -> ("YES"=w680:bool)  [unwired: 17 in, 1 out]
        "stop ok" <- w680
        n319 = property on="Tab Control" class="TabCtl (strict)"() -> ("Value"=w679:enum32{"Page 1", "Page 2", "Page 3"})  [unwired: 2 in, 2 out]
      }
      event "report": Value Change {
        n320 = event-data() -> ()  [unwired: 1 in, 6 out]
      }
    }
    "Tab Control" <- w670
    n321 = local write "stop tab control"(w673) -> ()
    n322 = Wait (ms)(milliseconds to wait=u32 10) -> ()  [unwired: 1 out]
  }
  "stop tab control" <- w92
  n323 = call "IMAQ Create"("Image Name"="img crop", "error in (no error)"=w48) -> ("New Image"=w55:T1, "error out"=w57:errorcluster)  [unwired: 3 in]
  n324 = local write "PLT NUM SYNC"(w90) -> ()
  n325 = local write "Sync"(w91) -> ()
  n326 = call "IMAQ Create"("Image Name"="pic2", "Image Type"=w100, "error in (no error)"=errorcluster {"status"=FALSE, "code"=0, "source"=""}) -> ("New Image"=w104:T1, "error out"=w103:errorcluster)  [unwired: 2 in]
  n327 = while {
    tunnel: w57 -> [w687]
    tunnel: [w683] -> w54
    stop <- w684 stop-if-true
    n328 = call "load Defects Script.vi"("error in (no error)"=w687) -> ("error out"=w683:errorcluster)  [unwired: 10 in]
    n329 = local read "stop ok"() -> (w685:bool)
    n330 = Not(x=w683) -> (.not. x?=w686:bool)
    n331 = Or(x=w686, y=w685) -> (x .or. y?=w684:bool)
  }
  n332 = while {
    tunnel: w37 -> [w786]
    shift-right: [w767] -> _
    shift-left: w31 -> [w783]
    shift-right: [w762] -> _
    shift-left: w30 -> [w780]
    shift-right: [w761] -> _
    shift-left: w29 -> [w778]
    shift-right: [w760] -> _
    shift-left: w28 -> [w776]
    shift-right: [w759] -> _
    shift-left: w27 -> [w774]
    tunnel: w26 -> [w772]
    shift-right: [w744] -> _
    shift-left: 0.0 ("element") -> [w758]
    tunnel: [w740] -> w24
    tunnel: [FALSE ("Col. Count")] -> w23
    tunnel: [FALSE ("Plt Count")] -> w22
    tunnel: w21 -> [w722]
    tunnel: [w720] -> w20
    shift-right: [w696] -> w19
    shift-left: w18 -> [w785]
    stop <- w720 stop-if-true
    # "coloumn counting"
    n333 = flat-sequence {
      tunnel: w786 -> [w811]
      tunnel: w785 -> [w810]
      tunnel: [w803] -> w784
      tunnel: w783 -> [w802]
      tunnel: [w802] -> w782
      tunnel: [w801] -> w781
      tunnel: w780 -> [w801]
      tunnel: [w800] -> w779
      tunnel: w778 -> [w800]
      tunnel: [w799] -> w777
      tunnel: w776 -> [w799]
      tunnel: [w798] -> w775
      tunnel: w774 -> [w798]
      tunnel: [w797] -> w773
      tunnel: w772 -> [w797]
      tunnel: [w789] -> w771
      tunnel: [w792] -> w770
      tunnel: w758 -> [w796]
      tunnel: [w796] -> w756
      tunnel: [w795] -> w741
      tunnel: [w794] -> w724
      tunnel: [w791] -> w723
      tunnel: w722 -> [w791]
      tunnel: w784 -> [w837]
      tunnel: w782 -> [w836]
      tunnel: w781 -> [w835]
      tunnel: w779 -> [w834]
      tunnel: w777 -> [w833]
      tunnel: w775 -> [w832]
      tunnel: w773 -> [w821]
      tunnel: w771 -> [w831]
      tunnel: w770 -> [w830]
      tunnel: [w817] -> w769
      tunnel: [w818] -> w768
      tunnel: [w829] -> w766
      tunnel: [w828] -> w765
      tunnel: [w827] -> w764
      tunnel: [w826] -> w763
      tunnel: [w825] -> w757
      tunnel: w756 -> [w825]
      tunnel: [w824] -> w755
      tunnel: [w823] -> w742
      tunnel: w741 -> [w823]
      tunnel: w724 -> [w822]
      tunnel: w723 -> [w820]
      tunnel: w769 -> [w857]
      tunnel: w768 -> [w864]
      tunnel: w766 -> [w863]
      tunnel: w765 -> [w862]
      tunnel: w764 -> [w861]
      tunnel: w763 -> [w860]
      tunnel: w757 -> [w858]
      tunnel: w755 -> [w840]
      tunnel: [w864] -> w754
      tunnel: [w863] -> w753
      tunnel: [w862] -> w752
      tunnel: [w861] -> w751
      tunnel: [w860] -> w750
      tunnel: [w857] -> w749
      tunnel: [w856] -> w748
      tunnel: [w846] -> w747
      tunnel: [w855] -> w746
      tunnel: [w854] -> w745
      tunnel: [w853] -> w743
      tunnel: w742 -> [w853]
      tunnel: [w852] -> w738
      tunnel: "capture" -> [w850]
      tunnel: [w843] -> w734
      tunnel: [w842] -> w733
      tunnel: w738 -> [w872]
      tunnel: w743 -> [w876]
      tunnel: "capture" -> [w875]
      tunnel: w745 -> [w873]
      tunnel: w746 -> [w874]
      tunnel: w747 -> [_]
      tunnel: w748 -> [w877]
      tunnel: w749 -> [w870]
      tunnel: w750 -> [w879]
      tunnel: w751 -> [w880]
      tunnel: w752 -> [w881]
      tunnel: w753 -> [w882]
      tunnel: w754 -> [w883]
      tunnel: w734 -> [w869]
      tunnel: w733 -> [w868]
      tunnel: [w883] -> w719
      tunnel: [w882] -> w717
      tunnel: [w881] -> w715
      tunnel: [w880] -> w713
      tunnel: [w879] -> w711
      tunnel: [w871] -> w709
      tunnel: [w873] -> w707
      tunnel: [w876] -> w705
      tunnel: [w868] -> w703
      tunnel: [w868] -> w701
      tunnel: w719 -> [w895]
      tunnel: [w895] -> w718
      tunnel: w717 -> [w894]
      tunnel: [w894] -> w716
      tunnel: w715 -> [w893]
      tunnel: [w893] -> w714
      tunnel: w713 -> [w892]
      tunnel: [w892] -> w712
      tunnel: w711 -> [w891]
      tunnel: [w891] -> w710
      tunnel: w709 -> [w890]
      tunnel: [w890] -> w708
      tunnel: w707 -> [w889]
      tunnel: [w889] -> w706
      tunnel: w705 -> [w888]
      tunnel: [w888] -> w704
      tunnel: w703 -> [w887]
      tunnel: [w887] -> w702
      tunnel: w701 -> [w884]
      tunnel: w718 -> [w908]
      tunnel: w716 -> [w907]
      tunnel: w714 -> [w906]
      tunnel: w712 -> [w905]
      tunnel: w710 -> [w904]
      tunnel: w708 -> [w903]
      tunnel: w706 -> [w902]
      tunnel: w704 -> [w901]
      tunnel: [w908] -> w732
      tunnel: [w907] -> w731
      tunnel: [w906] -> w730
      tunnel: [w905] -> w729
      tunnel: [w904] -> w728
      tunnel: [w903] -> w727
      tunnel: [w902] -> w726
      tunnel: [w901] -> w725
      tunnel: w702 -> [w900]
      tunnel: [w900] -> w721
      tunnel: w721 -> [w912]
      tunnel: w725 -> [w913]
      tunnel: w726 -> [w914]
      tunnel: w727 -> [w915]
      tunnel: w728 -> [w916]
      tunnel: w729 -> [w917]
      tunnel: w730 -> [w918]
      tunnel: w731 -> [w919]
      tunnel: w732 -> [w920]
      tunnel: [w920] -> w695
      tunnel: [w919] -> w694
      tunnel: [w918] -> w693
      tunnel: [w917] -> w692
      tunnel: [w916] -> w691
      tunnel: [w915] -> w690
      tunnel: [w914] -> w689
      tunnel: [w913] -> w688
      tunnel: [w922] -> w740
      tunnel: [w923] -> w696
      tunnel: [w924] -> w744
      tunnel: [w925] -> w759
      tunnel: [w926] -> w760
      tunnel: [w927] -> w761
      tunnel: [w928] -> w762
      tunnel: [w929] -> w767
      tunnel: w695 -> [w929]
      tunnel: w694 -> [w928]
      tunnel: w693 -> [w927]
      tunnel: w692 -> [w926]
      tunnel: w691 -> [w925]
      tunnel: w690 -> [w924]
      tunnel: w689 -> [w923]
      tunnel: w688 -> [w922]
      frame #0 {
        n334 = disable-structure shown="Disabled" {
          disable-tunnel: w811 -> [w816 _]
          disable-tunnel: w810 -> [w815 _]
          disable-tunnel: [w814 _] -> _
          disable-tunnel: [w813 _] -> w795
          disable-tunnel: [w812 _] -> w793
          frame Disabled {
            n335 = call "adamread.vi"("TCP Connection Refnum in"=w816, "error in (no error)"=w815) -> ("TCP Connection Refnum (dup)"=w813:refnum<k5>, "Slave Input Registers 2"=w814:dbl[], "error out 2"=w812:errorcluster)  [unwired: 11 in]
          }
          frame Enabled {
          }
        }
        n336 = local read "ch sensor1"() -> (w804:dbl)
        n337 = local read "ch sensor2"() -> (w805:dbl)
        n338 = local read "ch sensor3"() -> (w806:dbl)
        n339 = local read "ch sw sensor1"() -> (w807:dbl)
        n340 = local read "ch sw sensor2"() -> (w808:dbl)
        n341 = property on="denois level array" class="Arr (strict)"(error in=w793) -> (error out=w792:errorcluster, "Value"=w794:dbl[])  [unwired: 1 in, 1 out]
        n342 = Bundle(cluster=T8 {"ch sensor1"=0.0, "ch sensor2"=0.0, "ch sensor3"=0.0, "ch sw sensor1"=0.0, "ch sw sensor2"=0.0}, "ch sensor1"=w804, "ch sensor2"=w805, "ch sensor3"=w806, "ch sw sensor1"=w807, "ch sw sensor2"=w808) -> (w803:T8)
        n343 = call "waveform simulation.vi"("Frequency"=0.1) -> ("appended array"=w789:dbl[])  [unwired: 10 in]
      }
      frame #1 {
        n344 = call "sensor averaging.vi"("sensor chanel cluster"=w837, "array"=w836, "array 2"=w835, "array 3"=w834, "array 4"=w833, "array 5"=w832, "avg win1"=w820, "avg win2"=w821, "array sensor in"=w831, "error in"=w830, "denois level array"=w822) -> ("error out"=w824:errorcluster, "output array"=w818:dbl[], "output array 2"=w829:dbl[], "output array 3"=w828:dbl[], "output array 4"=w827:dbl[], "output array 5"=w826:dbl[], "avg data array"=w817:dbl[], "orgin data"=→"orgin data":dbl[])  [unwired: 9 in]
      }
      frame #2 {
        n345 = local read "1st sensor thr"() -> (w865:u32)
        n346 = local read "2nd sensor thr"() -> (w866:u16)
        n347 = local read "capture or not?"() -> (w859:bool)
        n348 = local read "3rd sensor thr"() -> (w867:u16)
        n349 = local read "counting role"() -> (w847:T2)
        n350 = Build Array(w865, w866, w867) -> (w848:u32[])
        n351 = property on="falling level thr" class="DigNum (strict)"(error in=w840) -> (error out=w839:errorcluster, "Value"=w841:dbl)  [unwired: 1 in, 1 out]
        n352 = property on="Debounce Time" class="DigNum (strict)"() -> ("Value"=w838:dbl)  [unwired: 2 in, 2 out]
        n353 = call "sensor count.vi"("sensor thr array"=w848, "debounce time"=w838, "capture y or no ?"=w859, "sensor data"=w857, "counter input"=w858, "counting role"=w847, "error in"=w839, "falling level thr"=w841) -> ("machine pallet stop"=w843:bool, "column count"=w852:bool, "capture trigger"=w851:bool, "sensor counter"=w855:bool, "speed"=w846:dbl, "counter out"=w856:dbl, "pallet detect"=→"Plt Count":bool, "error out"=w854:errorcluster)
        "speed 2" <- w846
        n354 = Number To Fractional String(number=w846, precision (6)=i16 3) -> (F-format string=→"Speed (m/min)":string)  [unwired: 2 in]
        n355 = Or(x=w851, y=w850) -> (x .or. y?=w842:bool)
      }
      frame #3 {
        n356 = Select(t=0.0, s=w875, f=w877) -> (s? t:f=w871:dbl)
        "Col\n NUM" <- w871
        "sensor counter" <- w874
        "Col. Count" <- w872
        "avg data array" <- w870
        "Run/Stop" <- w869
        "capture triger" <- w868
      }
      frame #4 {
        n357 = case shown="True" w884 {
          tunnel: [w896 FALSE ("SWR 2")] -> w886
          tunnel: [w897 FALSE ("SWL 2")] -> w885
          frame False {
            n358 = local read "SWR 2"() -> (w896:bool)
            n359 = local read "SWL 2"() -> (w897:bool)
          }
          frame True {
          }
        }
        n360 = local write "SWL 2"(w885) -> ()
        n361 = local write "SWR 2"(w886) -> ()
      }
      frame #5 {
        n362 = local write "rotate"(w900) -> ()
      }
      frame #6 {
        n363 = Select(t=u32 20 ("milliseconds to wait"), s=w912, f=u32 0) -> (s? t:f=w909:u32)
        n364 = Wait (ms)(milliseconds to wait=w909) -> ()  [unwired: 1 out]
      }
      frame #7 {
        n365 = local write "rotate"(FALSE ("rotate")) -> ()
      }
    }
    n366 = case shown="True" "capture" {
      frame False {
      }
      frame True {
        n367 = property on="Sync" class="Bool (strict)"("Value"=FALSE ("Sync")) -> ()  [unwired: 2 in, 2 out]
        "capture or not?" <- TRUE ("Boolean")
      }
    }
    n368 = property on="Col. Count" class="Bool (strict)"() -> ("Value"=w700:bool)  [unwired: 2 in, 2 out]
    n369 = Select(t=T6."Disabled" ("Disabled"), s=w700, f=T6."Enabled" ("Disabled")) -> (s? t:f=w697:T6)
    n370 = property on="capture" class="Bool"("DisabledEnum"=w697) -> ()  [unwired: 2 in, 2 out]
    n371 = Wait (ms)(milliseconds to wait=u32 4) -> ()  [unwired: 1 out]
    n372 = local read "stop ok"() -> (w720:bool)
    "sensor error in" <- w696
  }
  "coloumn count stop" <- w20
  n373 = Initialize Array "info array"(0.0 ("element"), 232 ("dimension size"), 15 ("dimension size")) -> (w49:dbl[][])
  n374 = call "IMAQ Create"("Image Name"="img input") -> ("New Image"=w43:T1)  [unwired: 4 in, 1 out]
  n375 = while {
    tunnel: w104 -> [w943]
    tunnel: [w933] -> w63
    shift-right: [w932] -> _
    shift-left: w103 -> [w935]
    stop <- w933 stop-if-true
    # "show selected pallet"
    n376 = Get Date/Time In Seconds() -> (seconds since 1Jan1904=w940:timestamp)
    n377 = local read "bottum array"() -> (w946:bool[])
    n378 = Get Date/Time String(seconds (now)=w940, want seconds? (F)=TRUE) -> (date string=→"time&date":string, time string=→"time&date 2":string)  [unwired: 1 in]
    n379 = local read "initilized array"() -> (w948:i16[])
    n380 = Boolean To (0,1)(Boolean=w946) -> (0, 1=w950:i16[])
    n381 = Or Array Elements(Boolean array=w946) -> (logical OR=w945:bool)
    n382 = Multiply(x=w950, y=w948) -> (x*y=w949:i16[])
    n383 = property on="bt ref array" class="Arr (strict)"(error in=w935) -> (error out=w934:errorcluster, "Value"=w936:refnum<vi>[])  [unwired: 1 in, 1 out]
    n384 = Add Array Elements(numeric array=w949) -> (sum=w947:i16)
    n385 = case shown="True" w945 {
      tunnel: [w965 w966] -> w944
      tunnel: w947 -> [_ w971]
      tunnel: w936 -> [_ w970]
      tunnel: [w964 w967] -> w942
      tunnel: w934 -> [w964 w968]
      frame False {
        n386 = local read "BoolText.Text"() -> (w965:string)
      }
      frame True {
        n387 = Index Array(array=w970, index=w971) -> (element=w969:refnum<vi>)
        n388 = property class="Bool"(reference=w969, error in=w968) -> (error out=w967:errorcluster, "BoolText.Text"=w966:string)  [unwired: 1 out]
      }
    }
    "BoolText.Text" <- w944
    n389 = Wait (ms)(milliseconds to wait=u32 5) -> ()  [unwired: 1 out]
    n390 = property on="last difrence" class="DigNum (strict)"() -> ("Value"=w931:i16)  [unwired: 2 in, 2 out]
    n391 = property on="Sync" class="Bool (strict)"() -> ("Value"=w930:bool)  [unwired: 2 in, 2 out]
    n392 = case shown="True" w945 {
      tunnel: w944 -> [_ w963]
      tunnel: w943 -> [_ w961]
      tunnel: w942 -> [w951 w960]
      tunnel: [w951 w955] -> w932
      tunnel: w931 -> [_ w954]
      tunnel: w930 -> [_ w953]
      frame False {
      }
      frame True {
        n393 = property on="info array" class="Arr (strict)"() -> ("Value"=w952:dbl[][])  [unwired: 2 in, 2 out]
        n394 = local read "path image"() -> (w962:path)
        n395 = call "imgwindow.vi"("String"=w963, "File Path"=w962, "sync"=w953, "inf array"=w952, "Image 2"=w961, "error in (no error)"=w960, "last difrence"=w954) -> ("This VI"=w959:refnum<vi>, "error out"=w958:errorcluster)  [unwired: 11 in]
        n396 = invoke class="VI" method="FP.Open"(reference=w959, error in=w958, "Activate"=TRUE ("Activate?"), "State"=T9."Standard") -> (error out=w955:errorcluster)  [unwired: 1 in, 4 out]
      }
    }
    "img show error" <- w932
    n397 = local read "stop ok"() -> (w933:bool)
  }
  "selected pallet stop" <- w63
  n398 = while {
    shift-right: [w997] -> _
    shift-left: w105 -> [w999]
    shift-right: [w995] -> _
    shift-left: 0 ("index") -> [w996]
    tunnel: [w993] -> w64
    shift-right: [w992] -> w61
    shift-left: w107 -> [w998]
    shift-right: [w974] -> _
    shift-left: 0 -> [w991]
    tunnel: w55 -> [w990]
    tunnel: w54 -> [w989]
    tunnel: w47 -> [w987]
    shift-right: [w979] -> _
    shift-left: w49 -> [w988]
    tunnel: [w978] -> w46
    tunnel: [w977] -> w45
    tunnel: w43 -> [w973]
    stop <- w993 stop-if-true
    # "main loop (rotate, process, labeling, syncron)"
    n399 = local read "rotate"() -> (w972:bool)
    n400 = case shown="True" w972 {
      tunnel: w999 -> [w1060 w1190]
      tunnel: w998 -> [w1061 w1189]
      tunnel: [w1060 w1063] -> w997
      tunnel: w996 -> [w1062 w1188]
      tunnel: [w1062 w1183] -> w995
      tunnel: [w1061 w1178] -> w992
      tunnel: w991 -> [w1057 w1168]
      tunnel: w990 -> [w1058 w1162]
      tunnel: w989 -> [w1056 w1145]
      tunnel: w988 -> [w1059 w1134]
      tunnel: w987 -> [_ w1108]
      tunnel: [w1059 w1088] -> w981
      tunnel: [w1058 w1082] -> w978
      tunnel: [w1056 w1081] -> w976
      tunnel: [w1057 w1080] -> w974
      tunnel: w973 -> [_ w1068]
      frame False {
      }
      frame True {
        n401 = flat-sequence {
          tunnel: w1188 -> [w1199]
          tunnel: w1189 -> [w1200]
          tunnel: w1190 -> [w1201]
          tunnel: [w1201] -> w1187
          tunnel: [w1200] -> w1186
          tunnel: [w1199] -> w1185
          tunnel: [w1198] -> w1169
          tunnel: w1168 -> [w1198]
          tunnel: [w1197] -> w1163
          tunnel: w1162 -> [w1197]
          tunnel: [w1196] -> w1146
          tunnel: w1145 -> [w1196]
          tunnel: [w1195] -> w1135
          tunnel: w1134 -> [w1195]
          tunnel: w1108 -> [w1194]
          tunnel: [w1194] -> w1097
          tunnel: [w1193] -> w1069
          tunnel: w1068 -> [w1193]
          tunnel: [w1212] -> w1192
          tunnel: [w1209] -> w1191
          tunnel: w1187 -> [w1215]
          tunnel: w1186 -> [w1225]
          tunnel: w1185 -> [w1211]
          tunnel: [w1214] -> w1184
          tunnel: [w1208] -> w1177
          tunnel: [w1207] -> w1170
          tunnel: w1169 -> [w1207]
          tunnel: [w1206] -> w1164
          tunnel: w1163 -> [w1206]
          tunnel: w1146 -> [w1205]
          tunnel: w1135 -> [w1204]
          tunnel: [w1204] -> w1128
          tunnel: [w1203] -> w1098
          tunnel: w1097 -> [w1203]
          tunnel: w1069 -> [w1202]
          tunnel: [w1202] -> w1065
          tunnel: w1191 -> [w1268]
          tunnel: w1192 -> [w1274]
          tunnel: w1184 -> [w1267]
          tunnel: [w1274] -> w1182
          tunnel: [w1268] -> w1183
          tunnel: [w1267] -> w1179
          tunnel: w1177 -> [w1266]
          tunnel: [w1265] -> w1175
          tunnel: [w1264] -> w1171
          tunnel: w1170 -> [w1264]
          tunnel: [w1263] -> w1165
          tunnel: w1164 -> [w1263]
          tunnel: [w1262] -> w1148
          tunnel: [w1261] -> w1136
          tunnel: [w1260] -> w1129
          tunnel: w1128 -> [w1260]
          tunnel: [w1259] -> w1123
          tunnel: [w1258] -> w1099
          tunnel: w1098 -> [w1258]
          tunnel: [w1257] -> w1066
          tunnel: w1065 -> [w1257]
          tunnel: w1182 -> [w1289]
          tunnel: [w1289] -> w1181
          tunnel: [w1288] -> w1180
          tunnel: w1179 -> [w1288]
          tunnel: [w1286] -> w1176
          tunnel: w1175 -> [w1286]
          tunnel: [w1285] -> w1172
          tunnel: w1171 -> [w1285]
          tunnel: [w1284] -> w1166
          tunnel: w1165 -> [w1284]
          tunnel: [w1278] -> w1149
          tunnel: w1148 -> [w1278]
          tunnel: [w1283] -> w1137
          tunnel: w1136 -> [w1283]
          tunnel: [w1282] -> w1130
          tunnel: w1129 -> [w1282]
          tunnel: [w1281] -> w1124
          tunnel: w1123 -> [w1281]
          tunnel: [w1280] -> w1100
          tunnel: w1099 -> [w1280]
          tunnel: [w1279] -> w1067
          tunnel: w1066 -> [w1279]
          tunnel: [w1278] -> w1064
          tunnel: [w1318] -> w1178
          tunnel: [w1319] -> w1063
          tunnel: w1181 -> [w1319]
          tunnel: w1180 -> [w1318]
          tunnel: w1176 -> [w1291]
          tunnel: [w1315] -> w1174
          tunnel: [w1314] -> w1173
          tunnel: w1172 -> [w1314]
          tunnel: [w1313] -> w1167
          tunnel: w1166 -> [w1313]
          tunnel: [w1312] -> w1161
          tunnel: [w1311] -> w1160
          tunnel: [w1310] -> w1159
          tunnel: [w1310] -> w1158
          tunnel: [w1309] -> w1157
          tunnel: [w1308] -> w1156
          tunnel: [w1307] -> w1155
          tunnel: [w1306] -> w1154
          tunnel: [w1305] -> w1153
          tunnel: [w1304] -> w1150
          tunnel: w1149 -> [w1304]
          tunnel: [w1303] -> w1138
          tunnel: w1137 -> [w1303]
          tunnel: [w1302] -> w1131
          tunnel: w1130 -> [w1302]
          tunnel: [w1301] -> w1125
          tunnel: w1124 -> [w1301]
          tunnel: [w1300] -> w1101
          tunnel: w1100 -> [w1300]
          tunnel: w1067 -> [w1299]
          tunnel: w1064 -> [w1294]
          tunnel: w1174 -> [w1347]
          tunnel: w1173 -> [w1346]
          tunnel: w1167 -> [w1341]
          tunnel: w1161 -> [w1340]
          tunnel: w1160 -> [w1339]
          tunnel: w1159 -> [w1338]
          tunnel: w1158 -> [w1337]
          tunnel: w1157 -> [w1334]
          tunnel: w1156 -> [w1333]
          tunnel: w1155 -> [w1325]
          tunnel: w1154 -> [w1326]
          tunnel: w1153 -> [w1330]
          tunnel: [w1329] -> w1152
          tunnel: [w1328] -> w1151
          tunnel: w1150 -> [w1328]
          tunnel: [w1327] -> w1147
          tunnel: [w1326] -> w1143
          tunnel: [w1325] -> w1141
          tunnel: [w1324] -> w1139
          tunnel: w1138 -> [w1324]
          tunnel: [w1323] -> w1132
          tunnel: w1131 -> [w1323]
          tunnel: [w1322] -> w1126
          tunnel: w1125 -> [w1322]
          tunnel: [w1321] -> w1102
          tunnel: w1101 -> [w1321]
          tunnel: [w1320] -> w1074
          tunnel: w1152 -> [w1373]
          tunnel: w1151 -> [w1372]
          tunnel: w1147 -> [w1371]
          tunnel: [w1370] -> w1144
          tunnel: w1143 -> [w1370]
          tunnel: [w1369] -> w1142
          tunnel: w1141 -> [w1369]
          tunnel: [w1368] -> w1140
          tunnel: w1139 -> [w1368]
          tunnel: [w1367] -> w1133
          tunnel: w1132 -> [w1367]
          tunnel: [w1365] -> w1127
          tunnel: w1126 -> [w1363]
          tunnel: [w1366] -> w1122
          tunnel: [w1364] -> w1103
          tunnel: w1102 -> [w1364]
          tunnel: [w1363] -> w1092
          tunnel: [w1362] -> w1083
          tunnel: [w1361] -> w1075
          tunnel: w1074 -> [w1361]
          tunnel: w1144 -> [w1420]
          tunnel: w1142 -> [w1419]
          tunnel: w1140 -> [w1385]
          tunnel: w1133 -> [w1430]
          tunnel: w1127 -> [w1386]
          tunnel: w1122 -> [w1410]
          tunnel: [w1387] -> w1121
          tunnel: [w1386] -> w1120
          tunnel: [w1384] -> w1119
          tunnel: [w1383] -> w1118
          tunnel: [w1382] -> w1104
          tunnel: w1103 -> [w1382]
          tunnel: [w1381] -> w1093
          tunnel: w1092 -> [w1381]
          tunnel: [w1380] -> w1084
          tunnel: w1083 -> [w1380]
          tunnel: [w1379] -> w1076
          tunnel: w1075 -> [w1379]
          tunnel: w1121 -> [w1444]
          tunnel: w1120 -> [w1450]
          tunnel: w1119 -> [w1443]
          tunnel: w1118 -> [w1449]
          tunnel: [w1448] -> w1117
          tunnel: [w1447] -> w1116
          tunnel: [w1446] -> w1115
          tunnel: [w1444] -> w1113
          tunnel: [w1443] -> w1111
          tunnel: [w1442] -> w1109
          tunnel: [w1440] -> w1105
          tunnel: w1104 -> [w1440]
          tunnel: [w1439] -> w1094
          tunnel: w1093 -> [w1439]
          tunnel: [w1438] -> w1085
          tunnel: w1084 -> [w1438]
          tunnel: [w1437] -> w1077
          tunnel: w1076 -> [w1437]
          tunnel: w1117 -> [w1462]
          tunnel: w1116 -> [w1461]
          tunnel: w1115 -> [w1460]
          tunnel: [w1459] -> w1114
          tunnel: w1113 -> [w1459]
          tunnel: [w1458] -> w1112
          tunnel: w1111 -> [w1458]
          tunnel: [w1457] -> w1110
          tunnel: w1109 -> [w1457]
          tunnel: [w1456] -> w1106
          tunnel: w1105 -> [w1456]
          tunnel: [w1455] -> w1095
          tunnel: w1094 -> [w1455]
          tunnel: [w1454] -> w1089
          tunnel: [w1453] -> w1086
          tunnel: w1085 -> [w1453]
          tunnel: [w1452] -> w1078
          tunnel: w1077 -> [w1452]
          tunnel: w1063 -> [w1451]
          tunnel: w1114 -> [w1488]
          tunnel: w1112 -> [w1487]
          tunnel: w1110 -> [w1485]
          tunnel: [w1484] -> w1107
          tunnel: w1106 -> [w1484]
          tunnel: [w1483] -> w1096
          tunnel: w1095 -> [w1483]
          tunnel: [w1482] -> w1091
          tunnel: [w1481] -> w1090
          tunnel: w1089 -> [w1481]
          tunnel: [w1480] -> w1087
          tunnel: w1086 -> [w1480]
          tunnel: [w1479] -> w1079
          tunnel: w1078 -> [w1479]
          tunnel: w1107 -> [w1500]
          tunnel: w1096 -> [w1499]
          tunnel: w1091 -> [w1497]
          tunnel: w1090 -> [w1498]
          tunnel: w1087 -> [w1496]
          tunnel: w1079 -> [w1494]
          tunnel: [w1497] -> w1073
          tunnel: [w1496] -> w1072
          tunnel: [w1495] -> w1071
          tunnel: [w1494] -> w1070
          tunnel: [w1502] -> w1080
          tunnel: [w1503] -> w1081
          tunnel: [w1504] -> w1082
          tunnel: [w1505] -> w1088
          tunnel: w1073 -> [w1505]
          tunnel: w1072 -> [w1504]
          tunnel: w1071 -> [w1503]
          tunnel: w1070 -> [w1502]
          frame #0 {
          }
          frame #1 {
            n402 = for {
              tunnel: w1215 -> [w1252] mode=indexing
              tunnel: [w1256] -> w1217 mode=indexing
              tunnel: w1225 -> [w1251] mode=indexing
              tunnel: [w1249] -> w1223 mode=indexing
              tunnel: [w1255] -> w1221 mode=indexing
              tunnel: [w1253] -> w1219 mode=indexing
              n403 = property class="Bool"(reference=w1252, error in=w1251) -> (error out=w1250:errorcluster, "BoolText.Text"=w1256:string)  [unwired: 1 out]
              n404 = property class="Bool"(reference=w1252, error in=w1250) -> (error out=w1249:errorcluster, "Colors [4]"=w1255:cluster{u32, u32}[])  [unwired: 1 out]
              n405 = Index Array(array=w1255, index=0) -> (element=w1253:cluster{u32, u32})
            }
            n406 = Greater?(x=w1211, y=231) -> (0:w1210:bool)
            n407 = Rotate 1D Array(1:w1219, 2:1 ("n")) -> (0:w1218:cluster{u32, u32}[])
            n408 = Rotate 1D Array(1:w1217, 2:1 ("n")) -> (0:w1216:string[])
            n409 = for {
              tunnel: w1215 -> [w1248] mode=indexing
              tunnel: w1216 -> [w1247] mode=indexing
              tunnel: [w1246] -> w1213 mode=indexing
              tunnel: w1223 -> [w1245] mode=indexing
              tunnel: w1221 -> [w1243] mode=indexing
              tunnel: w1215 -> [w1244] mode=indexing
              tunnel: w1218 -> [w1242] mode=indexing
              tunnel: [w1238] -> w1214 mode=indexing
              n410 = property class="Bool"(reference=w1248, error in=w1245, "BoolText.Text"=w1247) -> (reference out=w1246:refnum<vi>, error out=w1239:errorcluster)
              n411 = Replace Array Subset(array=w1243, new element=w1242, index=0) -> (w1240:cluster{u32, u32}[])
              n412 = property class="Bool"(reference=w1244, error in=w1239, "Colors [4]"=w1240) -> (error out=w1238:errorcluster)  [unwired: 1 out]
            }
            "bt ref array" <- w1213
            n413 = case shown="False" w1210 {
              tunnel: [w1232 w1237] -> w1209
              tunnel: w1211 -> [w1230 w1237]
              tunnel: w1213 -> [w1231 w1236]
              tunnel: [w1228 w1236] -> w1212
              tunnel: [w1227 w1235] -> w1208
              tunnel: w1205 -> [w1226 w1235]
              frame False {
                n414 = Increment(x=w1230) -> (x+1=w1232:i32)
                n415 = Index Array(array=w1231, index=w1230) -> (element=w1234:refnum<vi>)
                n416 = property class="Bool"(reference=w1234, error in=w1226, "DisabledEnum"=T6."Enabled" ("Disabled")) -> (reference out=w1229:refnum<vi>, error out=w1227:errorcluster)
                n417 = Replace Array Subset(array=w1231, new element=w1229, index=w1230) -> (w1228:refnum<vi>[])
              }
              frame True {
              }
            }
          }
          frame #2 {
            w1270 = 232 ("y")
            n418 = Index Array(array=w1274, index=0) -> (element=w1276:refnum<vi>)
            n419 = property class="Bool"(reference=w1276, error in=w1266) -> (error out=w1265:errorcluster, "BoolText.Text"=w1277:string)  [unwired: 1 out]
            n420 = local read "dis plt number"() -> (w1271:i32)
            n421 = Decimal String To Number(string=w1277) -> (number=w1259:i32)  [unwired: 2 in, 1 out]
            "PLT NUM" <- w1259
            n422 = Add(x=w1259, y=w1271) -> (x+y=w1269:i32)
            n423 = Subtract(x=w1269, y=w1270) -> (x-y=w1272:i32)
            n424 = Greater?(x=w1269, y=w1270) -> (0:w1273:bool)
            n425 = Select(t=w1272, s=w1273, f=w1269) -> (s? t:f=w1261:i32)
            "Sen Plt\nNUM" <- w1261
            "Sensor Pallet NUM" <- w1261
            n426 = Number To Decimal String(number=w1259) -> (decimal integer string=w1262:string)  [unwired: 1 in]
            "PLT NUM :" <- w1262
          }
          frame #3 {
            "Proc" <- TRUE ("Proc")
          }
          frame #4 {
            n427 = Concatenate Strings("E:\\arshad\\folad projects\\pallet car\\sirjan project\\DPIS\\pics\\" ("string"), "pallet(" ("string"), w1294, ").bmp" ("string")) -> (w1297:string)
            n428 = String To Path(string=w1297) -> (path=w1298:path)
            n429 = local read "threshoulds"() -> (w1317:dbl[])
            n430 = call "IMAQ ReadFile 2"("File Path"=w1298, "error in (no error)"=w1291, "Image"=w1299) -> ("error out"=w1290:errorcluster, "Image Out"=w1292:T1)  [unwired: 4 in, 3 out]
            n431 = call "wmlf Defects Script.vi"("threshoulds"=w1317, "margin"=dbl[] [650.0, 1550.0], "Image 3"=w1292, "error in (no error)"=w1290) -> ("function return"=w1315:i32, "x-y defects locs"=w1311:dbl[][], "defnum"=w1310:dbl, "def type"=w1307:dbl, "frame situation"=w1309:dbl, "obj num"=w1308:dbl, "def ratio"=w1306:dbl, "crop array"=w1312:dbl[][], "error out"=w1305:errorcluster)  [unwired: 15 in]
          }
          frame #5 {
            n432 = Equal To 0?(x=w1347) -> (x = 0?=w1348:bool)
            n433 = Greater Than 0?(x=w1337) -> (x > 0?=w1343:bool)
            n434 = call "IMAQ ArrayToImage"("error in (no error)"=w1330, "Image Pixels (U8)"=w1340, "Image"=w1341) -> ("error out"=w1344:errorcluster, "Image Out"=w1345:T1)  [unwired: 7 in]
            n435 = property on="Frame False Thr" class="DigNum (strict)"() -> ("Value"=w1332:dbl)  [unwired: 2 in, 2 out]
            n436 = case shown="True" w1348 {
              tunnel: w1346 -> [w1358 w1360]
              tunnel: [w1358 w1359] -> w1320
              frame False {
              }
              frame True {
                n437 = Increment(x=w1360) -> (x+1=w1359:i32)
              }
            }
            "nan error num" <- w1320
            n438 = local read "size"() -> (w1342:dbl)
            n439 = Equal To 0?(x=w1334) -> (x = 0?=w1336:bool)
            n440 = Less?(x=w1333, y=w1332) -> (x < y?=w1335:bool)
            n441 = case shown="True" w1343 {
              tunnel: w1345 -> [w1349 w1357]
              tunnel: w1344 -> [w1350 w1356]
              tunnel: [w1350 w1355] -> w1327
              tunnel: [w1349 w1354] -> w1329
              tunnel: w1339 -> [_ w1353]
              tunnel: w1342 -> [_ w1352]
              tunnel: w1338 -> [_ w1351]
              frame False {
              }
              frame True {
                n442 = call "bboxsubvi.vi"("Image"=w1357, "size"=w1352, "def num"=w1351, "array"=w1353, "error in"=w1356) -> ("Image Out"=w1354:T1, "error out"=w1355:errorcluster)  [unwired: 13 in]
              }
            }
            "Pallet Defects View" <- w1329
            n443 = Or(x=w1336, y=w1335) -> (x .or. y?=→"Frm False":bool)
            "GB defects%" <- w1326
            "DEF Type" <- w1325
          }
          frame #6 {
            # "indx 0 : GB defects\nindx 1 : Def Type\nindx 2 : GB sit\nindx 3 : curv\nindx 4 : curv sit\nindx 5 : swr\nindx 6 : swl\nindx 7 : pallet sit\nindx 8 : frm false\nindx 9 : sync\nindx 10 : col1 curv\nindx 11 : col2 curv\nindx 12 : col3 curv\nindx 13 : col4 curv\nindx 14 : col5 curv"
            n444 = local read "path image"() -> (w1376:path)
            n445 = Concatenate Strings("pallet_p(" ("string"), w1372, ").bmp" ("string")) -> (w1377:string)
            n446 = Build Path(base path=w1376, name or relative path=w1377) -> (appended path=w1378:path)
            n447 = Decrement(x=w1363) -> (x-1=w1365:i32)
            n448 = call-poly "IMAQ Write File 2"("error in (no error)"=w1371, "File Path"=w1378, "Image"=w1373) -> ("error out"=w1366:errorcluster, "Image Out (duplicate)"=w1362:T1)  [unwired: 7 in]
          }
          frame #7 {
            n449 = property on="Frm False" class="Bool (strict)"(error in=w1410) -> (error out=w1409:errorcluster, "Value"=w1408:bool)  [unwired: 1 in, 1 out]
            n450 = local read "2nd thr"() -> (w1432:dbl)
            n451 = property on="Sync" class="Bool (strict)"(error in=w1409) -> (error out=w1393:errorcluster, "Value"=w1406:bool)  [unwired: 1 in, 1 out]
            n452 = Boolean To (0,1)(Boolean=w1408) -> (0, 1=w1407:i16)
            n453 = local read "1st thr"() -> (w1433:dbl)
            n454 = property on="Col Curves" class="Arr (strict)"(error in=w1393) -> (error out=w1383:errorcluster, "Value"=w1394:dbl[])  [unwired: 1 in, 1 out]
            n455 = Boolean To (0,1)(Boolean=w1406) -> (0, 1=w1405:i16)
            n456 = Subtract(x=w1385, y=2) -> (x-y=w1436:i32)
            n457 = Less Than 0?(x=w1436) -> (x < 0?=w1435:bool)
            n458 = call "GB Situation.vi"("GB defects"=w1420, "def type"=w1419, "thr1"=w1433, "thr2"=w1432) -> ("GB sit"=w1418:i8)  [unwired: 11 in]
            n459 = local read "curv sit"() -> (w1416:bool)
            n460 = local read "SWR 2"() -> (w1414:bool)
            n461 = local read "SWL 2"() -> (w1412:bool)
            n462 = local read "CURV (mm)"() -> (w1417:dbl)
            n463 = Select(t=i16 231, s=w1435, f=w1436) -> (s? t:f=w1384:i32)
            "sen plt indx" <- w1384
            n464 = Index Array(array=w1394, index #1=0 ("index"), index #2=1 ("index"), index #3=2 ("index"), index #4=3 ("index"), index #5=4 ("index")) -> (element #1=w1392:dbl, element #2=w1391:dbl, element #3=w1390:dbl, element #4=w1389:dbl, element #5=w1388:dbl)
            n465 = Boolean To (0,1)(Boolean=w1416) -> (0, 1=w1415:i16)
            n466 = Boolean To (0,1)(Boolean=w1414) -> (0, 1=w1413:i16)
            n467 = Boolean To (0,1)(Boolean=w1412) -> (0, 1=w1411:i16)
            n468 = Replace Array Subset(array=w1430, new element #1=w1420, index (row) #1=w1386, index (col) #1=0 ("disabled index (col)"), new element #2=w1419, index (row) #2=w1386, index (col) #2=1 ("disabled index (col)"), new element #3=w1418, index (row) #3=w1386, index (col) #3=2 ("disabled index (col)"), new element #4=w1417, index (row) #4=w1384, index (col) #4=3 ("disabled index (col)"), new element #5=w1415, index (row) #5=w1384, index (col) #5=4 ("disabled index (col)"), new element #6=w1413, index (row) #6=w1384, index (col) #6=5 ("disabled index (col)"), new element #7=w1411, index (row) #7=w1384, index (col) #7=6 ("disabled index (col)"), new element #8=w1407, index (row) #8=w1386, index (col) #8=8 ("disabled index (col)"), new element #9=w1405, index (row) #9=w1386, index (col) #9=9 ("disabled index (col)"), new element #10=w1392, index (row) #10=w1384, index (col) #10=10 ("disabled index (col)"), new element #11=w1391, index (row) #11=w1384, index (col) #11=11 ("disabled index (col)"), new element #12=w1390, index (row) #12=w1384, index (col) #12=12 ("disabled index (col)"), new element #13=w1389, index (row) #13=w1384, index (col) #13=13 ("disabled index (col)"), new element #14=w1388, index (row) #14=w1384, index (col) #14=14 ("disabled index (col)")) -> (w1387:dbl[][])
          }
          frame #8 {
            n469 = call "pallet labeling.vi"("info array"=w1444, "pallet num"=w1450, "curv num"=w1443, "error in (no error)"=w1449) -> ("curv plt color"=w1448:cluster{u32, u32}, "pallet colour"=w1447:cluster{u32, u32}, "pallet_sit"=w1442:i8, "alarm"=→"alarm":bool, "Color Box"=→"GB sit":u32, "error out"=w1446:errorcluster)  [unwired: 17 in, 1 out]
          }
          frame #9 {
            n470 = property on="bt ref array" class="Arr (strict)" props=["Value"](error in=w1460) -> (error out=w1467:errorcluster)  [unwired: 1 in, 2 out]
            n471 = Index Array(array=w1451, index #1=0 ("index"), index #2=188 ("index")) -> (element #1=w1474:refnum<vi>, element #2=w1469:refnum<vi>)
            n472 = property class="Bool"(reference=w1469, error in=w1467) -> (reference out=w1473:refnum<vi>, error out=w1472:errorcluster, "Colors [4]"=w1471:cluster{u32, u32}[])
            n473 = Replace Array Subset(array=w1471, new element=w1462, index=0) -> (w1470:cluster{u32, u32}[])
            n474 = property class="Bool"(reference=w1473, error in=w1472, "Colors [4]"=w1470) -> (error out=w1468:errorcluster)  [unwired: 1 out]
            n475 = property class="Bool"(reference=w1474, error in=w1468) -> (reference out=w1475:refnum<vi>, error out=w1476:errorcluster, "Colors [4]"=w1477:cluster{u32, u32}[])
            n476 = Replace Array Subset(array=w1477, new element=w1461, index=0) -> (w1478:cluster{u32, u32}[])
            n477 = property class="Bool"(reference=w1475, error in=w1476, "Colors [4]"=w1478) -> (error out=w1454:errorcluster)  [unwired: 1 out]
          }
          frame #10 {
            n478 = Replace Array Subset(array=w1488, new element=w1485, index (row)=w1487, index (col)=7 ("disabled index (col)")) -> (w1482:dbl[][])
          }
          frame #11 {
            n479 = property on="Sync" class="Bool (strict)"() -> ("Value"=w1491:bool)  [unwired: 2 in, 2 out]
            n480 = property on="Frm False" class="Bool (strict)"() -> ("Value"=w1492:bool)  [unwired: 2 in, 2 out]
            n481 = property on="Run/Stop" class="Bool (strict)"() -> ("Value"=w1489:bool)  [unwired: 2 in, 2 out]
            n482 = property on="Tabe name" class="Str"() -> ("Value"=w1493:string)  [unwired: 2 in, 2 out]
            n483 = Compound Arithmetic op=AND(w1491, invert w1492, invert w1489) -> (w1490:bool)
            n484 = call "pallet DB.vi"("pallet_num"=w1499, "connection reference"=w1500, "info array"=w1497, "Table"=w1493, "set data"=w1490, "error in"=w1498) -> ("error out"=w1495:errorcluster)  [unwired: 20 in, 1 out]
          }
          frame #12 {
            n485 = property on="Proc" class="Bool (strict)"("Value"=FALSE ("Proc")) -> ()  [unwired: 2 in, 2 out]
          }
        }
      }
    }
    n486 = Wait (ms)(milliseconds to wait=u32 5) -> ()  [unwired: 1 out]
    n487 = Boolean To (0,1)(Boolean="Refresh Button") -> (0, 1=w986:i16)
    n488 = Build Array(w986) -> (w985:i16[])
    n489 = Bundle By Name("Y"=w985) -> (w984:waveform(i16))  [unwired: 1 in]
    n490 = call-poly <vilib>:"Basic Level Trigger Detection.vi"("signal in"=w984, "level"=0.5, "error in (no error)"=w976) -> ("trigger detected?"=w983:bool, "error out"=w975:errorcluster)  [unwired: 10 in, 1 out]
    n491 = case shown="True" w983 {
      tunnel: "Refresh Button" -> [_ w1004]
      tunnel: [w1001 w1009] -> w979
      tunnel: w981 -> [w1001 w1006]
      tunnel: [w1000 w1003] -> w977
      tunnel: w975 -> [w1000 w1002]
      frame False {
      }
      frame True {
        n492 = local read "bottum refrence"() -> (w1012:refnum<vi>[])
        n493 = property on="PLT NUM" class="DigNum (strict)"() -> ("Value"=w1011:i16)  [unwired: 2 in, 2 out]
        n494 = In Range and Coerce(upper limit=i16 232 ("y"), x="PLT NUM SYNC", lower limit=i16 1) -> (In Range?=w1013:bool)  [unwired: 1 out]
        n495 = Subtract(x="PLT NUM SYNC", y=w1011) -> (x-y=w1010:i16)
        n496 = case shown="True" w1004 {
          tunnel: w1010 -> [_ w1014]
          frame False {
          }
          frame True {
            "last difrence" <- w1014
          }
        }
        n497 = case shown="True" w1013 {
          tunnel: w1012 -> [_ w1027]
          tunnel: "PLT NUM SYNC" -> [_ w1028]
          tunnel: w1010 -> [_ w1025]
          tunnel: [w1017 w1022] -> w1003
          tunnel: [w1015 w1021] -> w1009
          tunnel: w1006 -> [w1015 w1020]
          tunnel: w1002 -> [w1016 w1019]
          frame False {
            n498 = call "Display Message to User2"("error in (no error)"=w1016, "Enable"=TRUE) -> ("error out"=w1017:errorcluster)  [unwired: 8 in, 1 out]
          }
          frame True {
            n499 = for {
              tunnel: w1027 -> [w1055] mode=indexing
              tunnel: w1028 -> [w1050]
              tunnel: [w1046] -> w1023 mode=indexing
              tunnel: w1020 -> [w1045] mode=indexing
              tunnel: [w1042] -> w1024 mode=indexing
              tunnel: w1019 -> [w1040]
              i -> [w1044]
              n500 = Replace Array Subset(array=w1045, new element=0.0 ("new element/subarray"), index=9) -> (w1042:dbl[])
              n501 = Subtract(x=w1050, y=w1044) -> (x-y=w1047:i32)
              n502 = Less Or Equal?(x=w1047, y=0.0) -> (x <= y?=w1054:bool)
              n503 = Add(x=232.0, y=w1047) -> (x+y=w1048:dbl)
              n504 = Select(t=w1048, s=w1054, f=w1047) -> (s? t:f=w1053:dbl)
              n505 = Number To Decimal String(number=w1053) -> (decimal integer string=w1052:string)  [unwired: 1 in]
              n506 = property class="Bool"(reference=w1055, error in=w1040, "BoolText.Text"=w1052) -> (error out=w1046:errorcluster)  [unwired: 1 out]
            }
            n507 = for {
              N: 15 -> [_]
              shift-right: [w1031] -> w1021
              shift-left: w1024 -> [w1032]
              tunnel: [w1030] -> w1022
              tunnel: w1023 -> [w1030] mode=indexing
              tunnel: w1025 -> [w1029]
              i -> [w1034]
              n508 = Array Subset(array=w1032, index (row)=0 ("index"), index (col)=w1034, length (col)=1 ("length")) -> (w1037:dbl[][])  [unwired: 1 in]
              n509 = Reshape Array(w1037, 232 ("dimension size")) -> (w1035:dbl[])
              n510 = Rotate 1D Array(1:w1035, 2:w1029) -> (0:w1033:dbl[])
              n511 = Replace Array Subset(array=w1032, new element=w1033, index (col)=w1034) -> (w1031:dbl[][])  [unwired: 1 in]
            }
          }
        }
        "Sync" <- w1004
      }
    }
    "info array" <- w979
    n512 = local read "stop ok"() -> (w993:bool)
  }
  n513 = Initialize Array(0.0 ("element"), 232 ("dimension size"), 6 ("dimension size"), 5 ("dimension size")) -> (w5:dbl[][][])
  n514 = Initialize Array(0.0 ("element"), 250 ("dimension size")) -> (w4:dbl[])
  n515 = Initialize Array(0.0 ("element"), 250 ("dimension size")) -> (w1:dbl[])
  n516 = Initialize Array(0.0 ("element"), 6 ("dimension size")) -> (w3:dbl[])
  n517 = Initialize Array(0.0 ("element"), 250 ("dimension size")) -> (w2:dbl[])
  n518 = while {
    tunnel: [w1593] -> w65
    shift-right: [w1551] -> _
    shift-left: errorcluster {"status"=FALSE, "code"=0, "source"=""} ("error constant") -> [w1552]
    shift-right: [w1518] -> _
    shift-left: w5 -> [w1523]
    shift-right: [w1517] -> _
    shift-left: w4 -> [w1522]
    shift-right: [w1516] -> _
    shift-left: w3 -> [w1521]
    shift-right: [w1515] -> _
    shift-left: w2 -> [w1520]
    shift-right: [w1514] -> _
    shift-left: w1 -> [w1519]
    stop <- w1593 stop-if-true
    # "setting page"
    n519 = call "password.vi"("error in (no error)"=w1552) -> ("result"=w1566:bool, "This VI"=w1567:refnum<vi>, "error out"=w1564:errorcluster)  [unwired: 11 in, 1 out]
    n520 = case shown="True" "setting" {
      tunnel: w1567 -> [_ w1628]
      tunnel: [w1623 w1625] -> w1565
      tunnel: w1564 -> [w1623 w1624]
      frame False {
      }
      frame True {
        n521 = invoke class="VI" method="FP.Open"(reference=w1628, error in=w1624, "Activate"=TRUE ("Activate?"), "State"=T9."Standard") -> (error out=w1625:errorcluster)  [unwired: 1 in, 4 out]
      }
    }
    n522 = call "registration.vi"("Enable"=FALSE) -> ("Password"=w1512:string, "User Name"=w1511:string)  [unwired: 15 in, 2 out]
    n523 = property on="nan error num" class="DigNum (strict)"() -> ("Value"=w1553:i32)  [unwired: 2 in, 2 out]
    n524 = Equal?(x=w1512, y="DPIS") -> (x = y?=w1510:bool)
    n525 = Equal?(x=w1511, y="2020") -> (x = y?=w1509:bool)
    n526 = property on="all errors" class="Clust (strict)"() -> ("Value"=w1554:errorcluster)  [unwired: 2 in, 2 out]
    n527 = And(x=w1510, y=w1509) -> ()  [unwired: 1 out]
    n528 = call "setting page.vi"("NAN error"=w1553, "error constant"=w1554) -> ("sensor cluster"=w1607:T10, "This VI"=w1578:refnum<vi>, "grtbar"=w1577:T11, "curv cluster"=w1575:T12, "IP # 2"=→"IP #":string, "general setting"=w1601:T13, "counting role"=→"counting role":T2, "img path 2"=→"path image":path)  [unwired: 6 in]
    n529 = Unbundle By Name(w1575) -> ("Thr1"=w1592:dbl, "Thr2"=w1591:dbl, "Thr3"=w1590:dbl, "Port"=→"Remote Port":dbl, "time out"=→"timout":dbl, "SWR thr"=w1587:dbl, "SWL thr"=w1579:dbl, "Curv thr (mm)"=w1586:dbl, "SW timout(s)"=w1585:dbl, "falling level thr"=w1584:dbl, "denoise thr1"=w1583:dbl, "denoise thr2"=w1582:dbl, "denoise thr3"=w1581:dbl, "low level read thr"=w1580:dbl, "Debounce Time"=→"Debounce Time":dbl)
    "1st sensor thr" <- w1592
    "2nd sensor thr" <- w1591
    "3rd sensor thr" <- w1590
    "falling level thr" <- w1584
    n530 = case shown="True" w1566 {
      tunnel: w1578 -> [_ w1632]
      tunnel: w1565 -> [w1629 w1631]
      tunnel: [w1629 w1630] -> w1551
      frame False {
      }
      frame True {
        n531 = invoke class="VI" method="FP.Open"(reference=w1632, error in=w1631, "Activate"=TRUE ("Activate?"), "State"=T9."Standard") -> (error out=w1630:errorcluster)  [unwired: 1 in, 4 out]
      }
    }
    n532 = Unbundle By Name(w1577) -> ("level1 thr"=→"1st thr":dbl, "level2 thr"=→"2nd thr":dbl, "gr.th1"=w1620:dbl, "gr.th2"=w1619:dbl, "gr.th3"=w1618:dbl, "gr.th4"=w1617:dbl, "gr.th5"=w1616:dbl, "gr.th6"=w1615:dbl, "gr.th7"=w1614:dbl, "gr.th8"=w1613:dbl, "gr.th9"=w1612:dbl, "def size"=→"size":dbl, "Frame False Thr"=→"Frame False Thr":dbl)
    n533 = Unbundle By Name(w1601) -> ("plt number dis"=→"dis plt number":i16, "Table Name"=→"Tabe name":string, "Database Name"=→"database name":string, "DB days to save"=→"DB days to save":i16)
    n534 = Unbundle By Name(w1607) -> ("ch sensor1"=→"ch sensor1":dbl, "ch sensor2"=→"ch sensor2":dbl, "chs ensor3"=→"ch sensor3":dbl, "ch sw sensor1"=→"ch sw sensor1":dbl, "ch sw sensor2"=→"ch sw sensor2":dbl)
    n535 = property on="Frm False" class="Bool (strict)"() -> ("Value"=w1573:bool)  [unwired: 2 in, 2 out]
    n536 = property on="Run/Stop" class="Bool (strict)"() -> ("Value"=w1570:bool)  [unwired: 2 in, 2 out]
    n537 = Boolean To (0,1)(Boolean=w1573) -> (0, 1=w1572:i16)
    n538 = Boolean To (0,1)(Boolean=w1570) -> (0, 1=w1569:i16)
    n539 = Build Array(w1620, w1619, w1618, w1617, w1616, w1615, w1614, w1613, w1612) -> (→"threshoulds":dbl[])
    n540 = Build Array(w1587, w1586, w1585, w1579) -> (→"curv sw info":dbl[])
    n541 = Build Array(w1592, w1591, w1590, w1584, w1580, w1572, w1569) -> (→"sensor thr array":dbl[])
    n542 = Build Array(w1583, w1582, w1581) -> (→"denois level array":dbl[])
    n543 = local read "Col\n NUM"() -> (w1534:dbl)
    n544 = local read "capture or not?"() -> (w1535:bool)
    n545 = property on="img show error" class="Clust (strict)"() -> ("Value"=w1557:errorcluster)  [unwired: 2 in, 2 out]
    n546 = property on="camera error in" class="Clust (strict)"() -> ("Value"=w1556:errorcluster)  [unwired: 2 in, 2 out]
    n547 = property on="sensor error in" class="Clust (strict)"() -> ("Value"=w1561:errorcluster)  [unwired: 2 in, 2 out]
    n548 = property on="sensor error in" class="Clust (strict)"() -> ("Value"=w1558:errorcluster)  [unwired: 2 in, 2 out]
    n549 = property on="query error in" class="Clust (strict)"() -> ("Value"=w1560:errorcluster)  [unwired: 2 in, 2 out]
    n550 = property on="curv sw info" class="Arr (strict)"() -> ("Value"=w1531:dbl[])  [unwired: 2 in, 2 out]
    n551 = property on="avg data array" class="Arr (strict)"() -> ("Value"=w1530:dbl[])  [unwired: 2 in, 2 out]
    n552 = property on="sensor thr array" class="Arr (strict)"() -> ("Value"=w1532:dbl[])  [unwired: 2 in, 2 out]
    n553 = property on="counting role" class="Enum (strict)"() -> ("Value"=w1533:T2)  [unwired: 2 in, 2 out]
    n554 = property on="rotate error" class="Clust (strict)"() -> ("Value"=w1563:errorcluster)  [unwired: 2 in, 2 out]
    n555 = property on="rotate array" class="Arr (strict)"() -> ("Value"=w1562:errorcluster[])  [unwired: 2 in, 2 out]
    n556 = property on="alarm error" class="Clust (strict)"() -> ("Value"=w1559:errorcluster)  [unwired: 2 in, 2 out]
    n557 = property on="Sen Plt\nNUM" class="DigNum (strict)"() -> ("Value"=w1548:i16)  [unwired: 2 in, 2 out]
    n558 = Merge Errors(w1551, w1563, w1562, w1561, w1560, w1559, w1558, w1557, w1556) -> (→"all errors":errorcluster)
    n559 = call "Calibration page.vi"("sensor data array"=w1530, "sensor thr array"=w1532, "counting role"=w1533, "sensor1 array"=w1522, "curv array in"=w1521, "count in"=w1534, "sensor2 array"=w1520, "sensor3 array"=w1519, "curv sw info"=w1531, "capture"=w1535, "cyrv avg array in"=w1523, "sen plt num"=w1548) -> ("Left Sidewall"=→"SWL 2":bool, "cyrv avg array out"=w1518:dbl[][][], "Right Sidewall"=→"SWR 2":bool, "curv sit"=→"curv sit":bool, "Col Curve"=→"Col Curves":dbl[], "Curvness Sensors Graph"=→"Curvness Sensors Graph":dynamicdata, "SideWall Sensors Graph"=→"SideWall Sensors Graph":dynamicdata, "sensor1 array out"=w1517:dbl[], "curv array out"=w1516:dbl[], "sensor2 array out"=w1515:dbl[], "sensor3 array out"=w1514:dbl[], "Pallet CURV (mm)"=→"CURV (mm)" →"Overal CURV avg(mm)":dbl)  [unwired: 1 in, 3 out]
    n560 = local read "stop ok"() -> (w1593:bool)
    n561 = Array Subset(array=w1516, index=1) -> (w1540:dbl[])  [unwired: 1 in]
    n562 = Index Array(array=w1516, index #1=1 ("index"), index #2=2 ("index"), index #3=3 ("index"), index #4=4 ("index"), index #5=5 ("index")) -> (element #1=→"Col1 CURV(mm)":dbl, element #2=→"Col2 CURV(mm)":dbl, element #3=→"Col3 CURV(mm)":dbl, element #4=→"Col4 CURV(mm)":dbl, element #5=→"Col5 CURV(mm)":dbl)
    n563 = Array Max & Min(array=w1540) -> (max value=→"Overal CURV(mm)":dbl)  [unwired: 3 out]
    n564 = Wait (ms)(milliseconds to wait=u32 5) -> ()  [unwired: 1 out]
  }
  "setting stop" <- w65
  n565 = local write "Col. Count"(w23) -> ()
  n566 = local write "Plt Count"(w22) -> ()
  n567 = disable-structure shown="Disabled" {
    disable-tunnel: [w1637 _] -> w38
    disable-tunnel: w24 -> [w1636 _]
    disable-tunnel: w19 -> [w1635 _]
    frame Disabled {
      n568 = TCP Close Connection(connection ID=w1636, error in (no error)=w1635) -> (error out=w1637:errorcluster)  [unwired: 1 in, 1 out]
    }
    frame Enabled {
    }
  }
  "sensor error out" <- w38
  n569 = disable-structure shown="Disabled" {
    frame Disabled {
      n570 = while {
        tunnel: [w1653] -> w1639
        shift-right: [w1645] -> _
        shift-left: errorcluster {"status"=FALSE, "code"=0, "source"=""} ("error in (no error)") -> [w1646]
        stop <- w1653 stop-if-true
        # "ALARM loop"
        n571 = property on="alarm" class="Bool (strict)"() -> ("Value"=w1650:bool)  [unwired: 2 in, 2 out]
        n572 = Boolean To (0,1)(Boolean=w1650) -> (0, 1=w1652:i16)
        n573 = property on="SWL 2" class="Bool (strict)"() -> ("Value"=w1644:bool)  [unwired: 2 in, 2 out]
        n574 = property on="SWR 2" class="Bool (strict)"() -> ("Value"=w1643:bool)  [unwired: 2 in, 2 out]
        n575 = Build Array(w1652) -> (w1651:i16[])
        n576 = property on="sen plt indx" class="DigNum (strict)"() -> ("Value"=w1654:i32)  [unwired: 2 in, 2 out]
        n577 = Bundle By Name("Y"=w1651) -> (w1648:waveform(i16))  [unwired: 1 in]
        n578 = Or(x=w1644, y=w1643) -> (x .or. y?=w1642:bool)
        n579 = call-poly <vilib>:"Basic Level Trigger Detection.vi"("signal in"=w1648, "level"=0.5, "error in (no error)"=w1646) -> ("trigger detected?"=w1641:bool, "error out"=w1647:errorcluster)  [unwired: 10 in, 1 out]
        "alarm edge" <- w1641
        n580 = local read "PLT NUM"() -> (w1659:i16)
        n581 = case shown="True" "OFF" {
          tunnel: [errorcluster {"status"=FALSE, "code"=0, "source"=""} ("error out") w1671] -> w1662
          frame False {
          }
          frame True {
            n582 = local write "alarm"(FALSE ("alarm")) -> ()
            n583 = property on="Alarm" class="Bool (strict)"("Blinking"=FALSE) -> (error out=w1671:errorcluster)  [unwired: 2 in, 1 out]
          }
        }
        n584 = case shown="True" w1642 {
          tunnel: [errorcluster {"status"=FALSE, "code"=0, "source"=""} ("error out") w1678] -> w1661
          tunnel: path "C:/Users/Public/Music/Sample Music/alert_siren.wav" ("path") -> [_ w1677]
          frame False {
            n585 = local write "alarm"(FALSE ("alarm")) -> ()
          }
          frame True {
            n586 = call "alarm sound.vi"("path"=w1677) -> ("error out"=w1676:errorcluster)  [unwired: 10 in]
            n587 = property on="Alarm" class="Bool (strict)"(error in=w1676, "Blinking"=TRUE) -> (error out=w1678:errorcluster)  [unwired: 1 in, 1 out]
          }
        }
        n588 = call "defects text.vi"("pallet number"=w1659, "curv num"=w1654, "Start Button"=w1641, "error in"=w1647) -> ("This VI"=w1658:refnum<vi>, "error out"=w1657:errorcluster)  [unwired: 9 in, 1 out]
        n589 = Merge Errors(w1661, w1662, w1657) -> (w1660:errorcluster)
        n590 = case shown="True" "Sequence Button" {
          tunnel: w1658 -> [_ w1667]
          tunnel: w1660 -> [w1664 w1666]
          tunnel: [w1664 w1665] -> w1645
          frame False {
          }
          frame True {
            n591 = invoke class="VI" method="FP.Open"(reference=w1667, error in=w1666, "Activate"=TRUE ("Activate?"), "State"=T9."Standard") -> (error out=w1665:errorcluster)  [unwired: 1 in, 4 out]
          }
        }
        "alarm error" <- w1645
        n592 = local read "stop ok"() -> (w1653:bool)
        n593 = Wait (ms)(milliseconds to wait=u32 5) -> ()  [unwired: 1 out]
      }
      "alarm loop stop" <- w1639
    }
    frame Enabled {
    }
  }
  n594 = while {
    tunnel: [w1692] -> w40
    shift-right: [w1682] -> _
    shift-left: errorcluster {"status"=FALSE, "code"=0, "source"=""} ("error out") -> [w1696]
    stop <- w1692 stop-if-true
    # "QUERY loop"
    n595 = local read "Tabe name"() -> (w1684:string)
    n596 = local read "Proc"() -> (w1681:bool)
    n597 = Not(x=w1681) -> (.not. x?=w1694:bool)
    n598 = property on="database name" class="Str"() -> ("Value"=w1685:string)  [unwired: 2 in, 2 out]
    n599 = And(x="Search Button 2", y=w1694) -> (x .and. y?=w1693:bool)
    n600 = case shown="True" w1693 {
      tunnel: w1696 -> [w1740 w1762]
      tunnel: [w1740 w1763] -> w1691
      tunnel: [w1739 w1761] -> w1683
      tunnel: "UNTIL" -> [_ w1743]
      tunnel: "FROM" -> [_ w1744]
      tunnel: w1685 -> [_ w1742]
      tunnel: w1684 -> [_ w1741]
      frame False {
        n601 = local read "Table"() -> (w1739:string[][])
      }
      frame True {
        n602 = call "query.vi"("pallet number"="PALLET NUMBER", "pallet_num sel"="plt num sel", "TIME"="TIME", "time select"="time sel", "FROM"=w1744, "UNTIL"=w1743, "GB_SITUATION"="GB SITUATION", "GB_sit sel"="GB_sit sel", "DEFECTS_TYPE"="DEFECTS TYPE", "CURV_SITUATION"="CURV SITUATION", "def_type sel"="def type sel", "curv_sit sel"="curv sit sel", "SWR"="SWR", "SWL"="SWL", "SWR sel"="swr sel", "swl sel"="swl sel", "Pallet-sit"="PALLET SITUATION", "database name"=w1742, "pallet_sit sel"="pallet sit sel", "table name"=w1741, "error in (no error)"=w1762) -> ("Table"=w1761:string[][], "error out 2"=w1763:errorcluster)  [unwired: 5 in]
        "Table" <- w1761
      }
    }
    n603 = local read "Proc"() -> (w1680:bool)
    n604 = Not(x=w1680) -> (.not. x?=w1689:bool)
    n605 = And(x="Save As Button 2", y=w1689) -> (x .and. y?=w1688:bool)
    n606 = case shown="True" w1688 {
      tunnel: w1691 -> [w1698 w1737]
      tunnel: [w1698 w1701] -> w1682
      tunnel: w1683 -> [_ w1738]
      frame False {
      }
      frame True {
        n607 = Get Date/Time In Seconds() -> (seconds since 1Jan1904=w1732:timestamp)
        n608 = Seconds To Date/Time(time stamp (now)=w1732) -> (date time rec=w1731:T16)  [unwired: 1 in]
        n609 = Unbundle By Name(w1731) -> ("year"=w1730:i32, "month"=w1729:i32, "day of month"=w1728:i32, "hour"=w1727:i32, "minute"=w1726:i32, "second"=w1725:i32)
        n610 = Number To Decimal String(number=w1730, width (-)=i16 4) -> (decimal integer string=w1724:string)
        n611 = Number To Decimal String(number=w1729, width (-)=i16 2) -> (decimal integer string=w1722:string)
        n612 = Number To Decimal String(number=w1728, width (-)=i16 2) -> (decimal integer string=w1720:string)
        n613 = Number To Decimal String(number=w1727, width (-)=i16 2) -> (decimal integer string=w1718:string)
        n614 = Number To Decimal String(number=w1726, width (-)=i16 2) -> (decimal integer string=w1716:string)
        n615 = Number To Decimal String(number=w1725, width (-)=i16 2) -> (decimal integer string=w1714:string)
        n616 = Concatenate Strings("Report  " ("string"), w1724, "_" ("string"), w1722, "_" ("string"), w1720, "    " ("string"), w1718, ";" ("string"), w1716, ";" ("string"), w1714, ".xlsx" ("string")) -> (w1712:string)
        n617 = Build Path(base path="Base Path", name or relative path=w1712) -> (appended path=w1702:path)
        n618 = call <vilib>:"Create Report.vi"("window state (normal)"=T14."maximized", "report type"=Report_Type."Excel", "error in (no error)"=w1737) -> ("report out"=w1700:refnum<class "NI_report.lvclass">, "error out"=w1699:errorcluster)  [unwired: 11 in]
        n619 = property on="Table" class="Tbl (strict)"() -> ("Column Headers[]"=w1736:string[])  [unwired: 2 in, 2 out]
        n620 = call-poly <vilib>:"Excel Easy Table.vi"("report in"=w1700, "text data"=w1738, "error in (no error)"=w1699, "column headers"=w1736) -> ("report out"=w1703:refnum<class "NI_report.lvclass">, "error out"=w1704:errorcluster)  [unwired: 7 in, 3 out]
        n621 = call-dynamic "Save Report to File.vi"("report in"=w1703, "report file path"=w1702, "error in (no error)"=w1704) -> ("error out"=w1701:errorcluster)  [unwired: 11 in, 1 out]
      }
    }
    "query error in" <- w1682
    n622 = local read "stop ok"() -> (w1692:bool)
    n623 = Wait (ms)(milliseconds to wait=u32 10) -> ()  [unwired: 1 out]
  }
  "query stop" <- w40
  n624 = while {
    shift-right: [w1782] -> _
    shift-left: errorcluster {"status"=FALSE, "code"=0, "source"=""} ("error out") -> [w1783]
    stop <- w1786 stop-if-true
    # "Release a row of database after sum days (FIFO)"
    n625 = property on="database name" class="Str"() -> ("Value"=w1785:string)  [unwired: 2 in, 2 out]
    n626 = property on="Tabe name" class="Str"() -> ("Value"=w1784:string)  [unwired: 2 in, 2 out]
    n627 = property on="DB days to save" class="DigNum (strict)"() -> ("Value"=w1780:i16)  [unwired: 2 in, 2 out]
    n628 = call-poly <vilib>:"DB Tools Open Connection.vi"("error in (no error)"=w1783, "connection information"=w1785) -> ("error out"=w1766:errorcluster, "connection reference"=w1767:T7)  [unwired: 6 in]
    n629 = Multiply(x=u64 40000 ("y"), y=w1780) -> (x*y=w1779:u64)
    n630 = Get Date/Time In Seconds() -> (seconds since 1Jan1904=w1776:timestamp)
    n631 = To Unsigned Quad Integer(1:w1776) -> (0:w1777:u64)
    n632 = Multiply(x=u64 40 ("y"), y=w1780) -> (x*y=w1770:u64)
    n633 = Subtract(x=w1777, y=w1770) -> (x-y=w1778:u64)
    n634 = To Time Stamp(1:w1778) -> (0:w1769:timestamp)
    n635 = Wait (ms)(milliseconds to wait=w1779) -> ()  [unwired: 1 out]
    n636 = Format Date/Time String(time format string (%c)="%Y-%m-%d %H:%M:%S", seconds (now)=w1769) -> (date/time string=w1773:string)  [unwired: 1 in]
    n637 = Concatenate Strings("WHERE DATE_TIME < '" ("condition"), w1773, "'" ("condition")) -> (w1768:string)
    n638 = call <vilib>:"DB Tools Delete Data.vi"("condition"=w1768, "error in (no error)"=w1766, "table"=w1784, "connection reference"=w1767) -> ("error out"=w1764:errorcluster, "connection reference out"=w1765:T7)  [unwired: 6 in]
    n639 = call <vilib>:"DB Tools Close Connection.vi"("error in (no error)"=w1764, "connection reference"=w1765) -> ("error out"=w1782:errorcluster)  [unwired: 5 in]
    n640 = local read "stop ok"() -> (w1786:bool)
  }
  n641 = while {
    stop <- FALSE stop-if-true
    n642 = property on="coloumn count stop" class="Bool (strict)"() -> ("Value"=w1791:bool)  [unwired: 2 in, 2 out]
    n643 = Wait (ms)(milliseconds to wait=u32 20) -> ()  [unwired: 1 out]
    n644 = property on="selected pallet stop" class="Bool (strict)"() -> ("Value"=w1795:bool)  [unwired: 2 in, 2 out]
    n645 = property on="bottum loop stop" class="Bool (strict)"() -> ("Value"=w1792:bool)  [unwired: 2 in, 2 out]
    n646 = property on="stop tab control" class="Bool (strict)"() -> ("Value"=w1794:bool)  [unwired: 2 in, 2 out]
    n647 = property on="stop live view" class="Bool (strict)"() -> ("Value"=w1793:bool)  [unwired: 2 in, 2 out]
    n648 = property on="setting stop" class="Bool (strict)"() -> ("Value"=w1797:bool)  [unwired: 2 in, 2 out]
    n649 = property on="rotate stop" class="Bool (strict)"() -> ("Value"=w1796:bool)  [unwired: 2 in, 2 out]
    n650 = property on="query stop" class="Bool (strict)"() -> ("Value"=w1790:bool)  [unwired: 2 in, 2 out]
    n651 = Compound Arithmetic op=AND(w1797, w1796, w1795, w1794, w1793, w1792, w1791, w1790) -> (w1789:bool)
    n652 = Quit LabVIEW(quit? (T)=w1789) -> ()
  }
  n653 = call "IMAQ Dispose"("Image"=w46, "error in (no error)"=w45) -> ("error out"=→"process error out  2":errorcluster)  [unwired: 4 in]
  n654 = for {
    tunnel: w105 -> [w1805] mode=indexing
    tunnel: w61 -> [w1804] mode=indexing
    tunnel: [w1798] -> w66
    tunnel: w64 -> [w1798]
    n655 = property class="Bool"(reference=w1805, error in=w1804) -> (reference out=w1810:refnum<vi>, error out=w1808:errorcluster, "Label.Text"=w1809:string)
    n656 = control-ref of="Button"() -> (w1799:refnum<vi>)
    n657 = property class="Bool"(reference=w1810, error in=w1808, "BoolText.Text"=w1809) -> (reference out=w1802:refnum<vi>, error out=w1803:errorcluster)
    n658 = property class="Bool"(reference=w1799) -> ("Colors [4]"=w1806:cluster{u32, u32}[])  [unwired: 1 in, 2 out]
    n659 = property class="Bool"(reference=w1802, error in=w1803, "Colors [4]"=w1806) -> (reference out=w1801:refnum<vi>, error out=w1800:errorcluster)
    n660 = property class="Bool"(reference=w1801, error in=w1800, "DisabledEnum"=T6."Disabled and Grayed Out" ("Disabled")) -> ()  [unwired: 2 out]
  }
  "rotate stop" <- w66
  "ready" <- w67
  "rotate" <- w67
